vi "Vision_Right_R3.4.vi"() -> ()   [LabVIEW 2015]
uses:
  <vilib>/vision/driver/NI_Vision_Acquisition_Software.lvlib
  <vilib>/userdefined/High Color/IMAQdx.ctl
  <vilib>/vision/NI_Vision_Development_Module.lvlib
  <vilib>/vision/Pattern Matching.llb/IMAQ Match Range Setting.ctl
  <vilib>/vision/Pattern Matching.llb/IMAQ Curve Parameters.ctl
panel:
  in  "RIGHT ORIENTED\nSHARED VAR":bool
  out "LEFT ORIENTED\nSHARED VAR 2":bool
  out "STARTUP COMPLETE\nSHARED VAR":bool
  out "Facing South\nSHARED VAR":bool
  out "Found Template\nSHARED VAR":i32
  in  "StartCase Found - LEFT 2\nREAD SV":bool
  out "StartCase Found - LEFT\nSHARED VAR":bool
  in  "Min Corr Score\nStart":sgl
  out "Start Case\nCorrelation Score\nSHARED VAR":sgl
  in  "select (true= use advanced features\nfase= dont use) 2":bool
  in  "Start Template\nIndex":i32
  in  "Start Template \nFilePaths - ARRAY":path[](array[path])=[path "/home/lvuser/Beacon_Templates/Range_2/Sub 0 - Range 2.png", path "/home/lvuser/Beacon_Templates/Range_2/Sub 1 - Range 2.png", path "/home/lvuser/Beacon_Templates/Range_2/Sub 2 - Range 2.png", path "/home/lvuser/Beacon_Templates/Range_2/Sub 3 - Range 2.png", path "/home/lvuser/Beacon_Templates/Range_2/Sub 4 - Range 2.png"]
  in  "master Startup":bool=TRUE
  in  "Range 0 Default\nSetting Values":T1={"Min Scale"=50.0, "Max Scale"=160.0, "Min Score"=850.0, "Lower Transition Scale"=45.0, "Upper Transition Scale"=200.0, "ROI Vertical"=2.0, "ROI Horizontal"=1.0, "Scale Cushion"=15.0, "Curve Parameters"={"Min Length"=15, "Row Search Step"=10, "Col Search Step"=10}, "Beacon Cushion (px)"=3.0, "Max Scale Diff\nfrom Main"=50.0}
  in  "Range 0 Templates":T2={"Sub - 2 File Path"=path "/home/lvuser/Beacon_Templates/Range_0/Range 0.png", "Sub Beacon Template File Path - ARRAY"=[path "/home/lvuser/Beacon_Templates/Range_1/Sub 0 - Range 1.png", path "/home/lvuser/Beacon_Templates/Range_1/Sub 1 - Range 1.png", path "/home/lvuser/Beacon_Templates/Range_1/Sub 2 - Range 1.png", path "/home/lvuser/Beacon_Templates/Range_1/Sub 3 - Range 1.png", path "/home/lvuser/Beacon_Templates/Range_1/Sub 4 - Range 1.png"]}
  in  "Correlation Score Threhsold (Range 0)":sgl=750.0
  in  "stop":bool
  in  "select (true= use advanced features\nfase= dont use)":bool
  in  "Range 3 Default\nSetting Values":T1={"Min Scale"=50.0, "Max Scale"=150.0, "Min Score"=800.0, "Lower Transition Scale"=1.0, "Upper Transition Scale"=130.0, "ROI Vertical"=3.5, "ROI Horizontal"=4.0, "Scale Cushion"=15.0, "Curve Parameters"={"Min Length"=2, "Row Search Step"=5, "Col Search Step"=5}, "Beacon Cushion (px)"=5.0, "Max Scale Diff\nfrom Main"=10.0}
  in  "Range 2 Default\nSetting Values":T1={"Min Scale"=65.0, "Max Scale"=130.0, "Min Score"=800.0, "Lower Transition Scale"=65.0, "Upper Transition Scale"=125.0, "ROI Vertical"=2.8, "ROI Horizontal"=4.0, "Scale Cushion"=17.0, "Curve Parameters"={"Min Length"=10, "Row Search Step"=10, "Col Search Step"=10}, "Beacon Cushion (px)"=15.0, "Max Scale Diff\nfrom Main"=20.0}
  in  "No Lock Default\nSetting Values":T3={"Min Scale"=25.0, "Max Scale"=200.0, "Min Score"=750.0, "Lower Transition Scale"=35.0, "Upper Transition Scale"=250.0, "ROI Vertical"=15.0, "ROI Horizontal"=15.0, "Scale Cushion"=15.0, "Curve Parameters"={"Min Length"=5, "Row Search Step"=10, "Col Search Step"=10}, "Scale Cushion 2"=15.0, "Max Scale Diff\nfrom Main"=15.0}
  in  "ROI Decay Factor (px)":dbl=50.0
  in  "ROBOT STATE\n(fwd, bwd, neither) 2":i32
  in  "Score Decay \nFactor 2":dbl=50.0
  in  "Range 1 Default\nSetting Values":T1={"Min Scale"=25.0, "Max Scale"=100.0, "Min Score"=800.0, "Lower Transition Scale"=35.0, "Upper Transition Scale"=67.0, "ROI Vertical"=0.75, "ROI Horizontal"=5.0, "Scale Cushion"=23.0, "Curve Parameters"={"Min Length"=15, "Row Search Step"=15, "Col Search Step"=15}, "Beacon Cushion (px)"=25.0, "Max Scale Diff\nfrom Main"=25.0}
  out "Next Template":T4(ring)
  out "Current Template":T4(ring)
  in  "Initial Template":T4(ring)
  in  "Range 3 Templates":T2={"Sub - 2 File Path"=path "/home/lvuser/Beacon_Templates/Range_3/5 Beacons - Range 3.png", "Sub Beacon Template File Path - ARRAY"=[path "/home/lvuser/Beacon_Templates/Range_3/Sub 0 - Range 3.png", path "/home/lvuser/Beacon_Templates/Range_3/Sub 1 - Range 3.png", path "/home/lvuser/Beacon_Templates/Range_3/Sub 2 - Range 3.png", path "/home/lvuser/Beacon_Templates/Range_3/Sub 3 - Range 3.png", path "/home/lvuser/Beacon_Templates/Range_3/Sub 4 - Range 3.png"]}
  in  "Range 2 Templates":T2={"Sub - 2 File Path"=path "/home/lvuser/Beacon_Templates/Range_2/5 Beacons - Range 2.png", "Sub Beacon Template File Path - ARRAY"=[path "/home/lvuser/Beacon_Templates/Range_2/Sub 0 - Range 2.png", path "/home/lvuser/Beacon_Templates/Range_2/Sub 1 - Range 2.png", path "/home/lvuser/Beacon_Templates/Range_2/Sub 2 - Range 2.png", path "/home/lvuser/Beacon_Templates/Range_2/Sub 3 - Range 2.png", path "/home/lvuser/Beacon_Templates/Range_2/Sub 4 - Range 2.png"]}
  in  "Range 1 Templates - RIGHT":T2={"Sub - 2 File Path"=path "/home/lvuser/Beacon_Templates/Range_1/2_Beacons_Right - Range 1.png", "Sub Beacon Template File Path - ARRAY"=[path "/home/lvuser/Beacon_Templates/Range_1/Sub 0 - Range 1.png", path "/home/lvuser/Beacon_Templates/Range_1/Sub 1 - Range 1.png", path "/home/lvuser/Beacon_Templates/Range_1/Sub 2 - Range 1.png", path "/home/lvuser/Beacon_Templates/Range_1/Sub 3 - Range 1.png", path "/home/lvuser/Beacon_Templates/Range_1/Sub 4 - Range 1.png"]}
  out "Current Correlation Score":sgl
  in  "Correlation Score Threhsold":sgl=300.0
  out "New Min Score":dbl=800.0
  out "New Low Scale":dbl=25.0
  out "New high Scale":dbl=100.0
  in  "Absolute\nMinimum Score":dbl=750.0
  in  "Absolute\nMaximum Scale":dbl=250.0
  in  "Absolute\nMinimum Scale":dbl=25.0
  in  "Score\nCushion":dbl=192.0
  in  "Avg Scale - Last":dbl=50.0
  in  "Avg Score - Last":dbl=986.6820373535156
  in  "Max Window\n for Avg":u8=3
  in  "Valid Treshold\nfor Lock":i16=3
  out "Current  Score":sgl
  out "Current  Scale":sgl
  out "Current Valid?":bool
  out "Beacon - Scales":sgl[](array[numeric])
  out "beacon - Scores":sgl[](array[numeric])
  out "Beacons Found":bool[](array[boolean])
  out "Horiztonall Beacon \nCushion (pixels)":sgl=25.0
  out "Tracking Info":T5={"Lock"=FALSE, "Current Valid"=FALSE, "Current Template"=enum."Range 1", "Tracking Coordinates"={"X"=159.0, "Y"=119.0}, "Setting Values"={"Min Score"=800.0, "Min Scale"=25.0, "Max Scale"=100.0, "Curve Parameters"={"Min Length"=15, "Row Search Step"=15, "Col Search Step"=15}}}
  out "dT":u32=629
  out "Avg Scale":dbl=50.0
  out "Avg Score":dbl=986.6820373535156
  out "Current Search Settings":T8={"Curve Parameters"={"Extraction Mode"=1, "Edge Threshold"=200, "Edge Filter Size"=0, "Min Length"=15, "Row Search Step Size"=15, "Col Search Step Size"=15, "Max Endpoint Gap"=4, "Closed"=TRUE, "Subpixel"=TRUE}, "Match Mode"={"Rotation"=TRUE, "Scale"=TRUE, "Occlusion"=TRUE, "Reserved"=FALSE, "Reserved"=FALSE, "Reserved"=FALSE}, "Range Settings"=[{"Match Constraints"=0, "Min"=-10.0, "Max"=2.0}, {"Match Constraints"=1, "Min"=25.0, "Max"=100.0}, {"Match Constraints"=2, "Min"=0.0, "Max"=20.0}], "Number of Matches"=1, "Minimum Match Score"=800.0, "SubPixel Accuracy"=TRUE, "Adv. Geometric Match Options 2"=[{"Setup Data Item"=20, "Item Value"=0.0}, {"Setup Data Item"=22, "Item Value"=1.0}]} {"Curve Parameters"."Extraction Mode" items=["Normal", "Uniform Regions"]; "Curve Parameters"."Edge Filter Size" items=["Fine", "Normal", "Contour Tracing"]; "Curve Parameters"."Max Endpoint Gap" min=0; "Curve Parameters"."Col Search Step Size" min=1 max=255 step=1; "Curve Parameters"."Row Search Step Size" min=1 max=255 step=1; "Curve Parameters"."Min Length" min=0; "Curve Parameters"."Edge Threshold" min=1 max=350 step=1; "Range Settings"."Max" format="%.2f"; "Range Settings"."Min" format="%.2f"; "Range Settings"."Match Constraints" items=["Rotation Angle (degrees)", "Scale Factor (%)", "Occlusion (%)"]}
  out "Valid Scale History":dbl[](array[numeric]) format="%#_13g"
  out "Valid Score History":dbl[](array[numeric]) format="%#_13g"
  out "Valid Beacon History - in":bool[](array[boolean])
  out "Startup Flag":bool
  out "Lock Status":bool
  out "Y Coordinates":sgl[](array[numeric])
  out "X Coordinates":sgl[](array[numeric])
  out "Right Image out":T9(plugin-control)
  in  "History Size":i32=19
  in  "INITIAL Search Settings":T8={"Curve Parameters"={"Extraction Mode"=1, "Edge Threshold"=200, "Edge Filter Size"=0, "Min Length"=15, "Row Search Step Size"=10, "Col Search Step Size"=10, "Max Endpoint Gap"=4, "Closed"=TRUE, "Subpixel"=TRUE}, "Match Mode"={"Rotation"=TRUE, "Scale"=TRUE, "Occlusion"=TRUE, "Reserved"=FALSE, "Reserved"=FALSE, "Reserved"=FALSE}, "Range Settings"=[{"Match Constraints"=0, "Min"=-10.0, "Max"=2.0}, {"Match Constraints"=1, "Min"=25.0, "Max"=150.0}, {"Match Constraints"=2, "Min"=0.0, "Max"=20.0}], "Number of Matches"=1, "Minimum Match Score"=750.0, "SubPixel Accuracy"=TRUE, "Adv. Geometric Match Options 2"=[{"Setup Data Item"=20, "Item Value"=0.0}, {"Setup Data Item"=22, "Item Value"=1.0}]} {"Curve Parameters"."Extraction Mode" items=["Normal", "Uniform Regions"]; "Curve Parameters"."Edge Filter Size" items=["Fine", "Normal", "Contour Tracing"]; "Curve Parameters"."Max Endpoint Gap" min=0; "Curve Parameters"."Col Search Step Size" min=1 max=255 step=1; "Curve Parameters"."Row Search Step Size" min=1 max=255 step=1; "Curve Parameters"."Min Length" min=0; "Curve Parameters"."Edge Threshold" min=1 max=350 step=1; "Range Settings"."Max" format="%.2f"; "Range Settings"."Min" format="%.2f"; "Range Settings"."Match Constraints" items=["Rotation Angle (degrees)", "Scale Factor (%)", "Occlusion (%)"]; "Adv. Geometric Match Options 2"."Setup Data Item" items=["Curve Extraction Mode", "Curve Edge Threshold", "Curve Edge Filter Size", "Min Curve Length", "Curve Row Search Step Size", "Curve Col Search Step Size", "Curve Max Endpoint Gap", "Extract Closed Curves", "Enable Subpixel Curve Extraction", "Enable Correlation Score", "Enable Subpixel Accuracy", "Subpixel Iterations", "Subpixel Tolerance", "Initial Match List Length", "Enable Target Template Curve Score", "Min Match Separation Distance", "Min Match Separation Angle", "Min Match Separation Scale", "Max Match Overlap", "Enable Coarse Result", "Enable Calibration Support", "Enable Contrast Reversal", "Search Strategy", "Refinement Match Factor", "Subpixel Match Factor"]}
  # "ROI Factore (per Template)"
  # "Template Transition Scales"
  # "Search Parameter Limits"
  # "TEMPLATE FILE PATHS"
  # "Config"
  # "Initial Settings"
  # "STARTUP SPECIFIC"
  # "Range"
  # "Range"
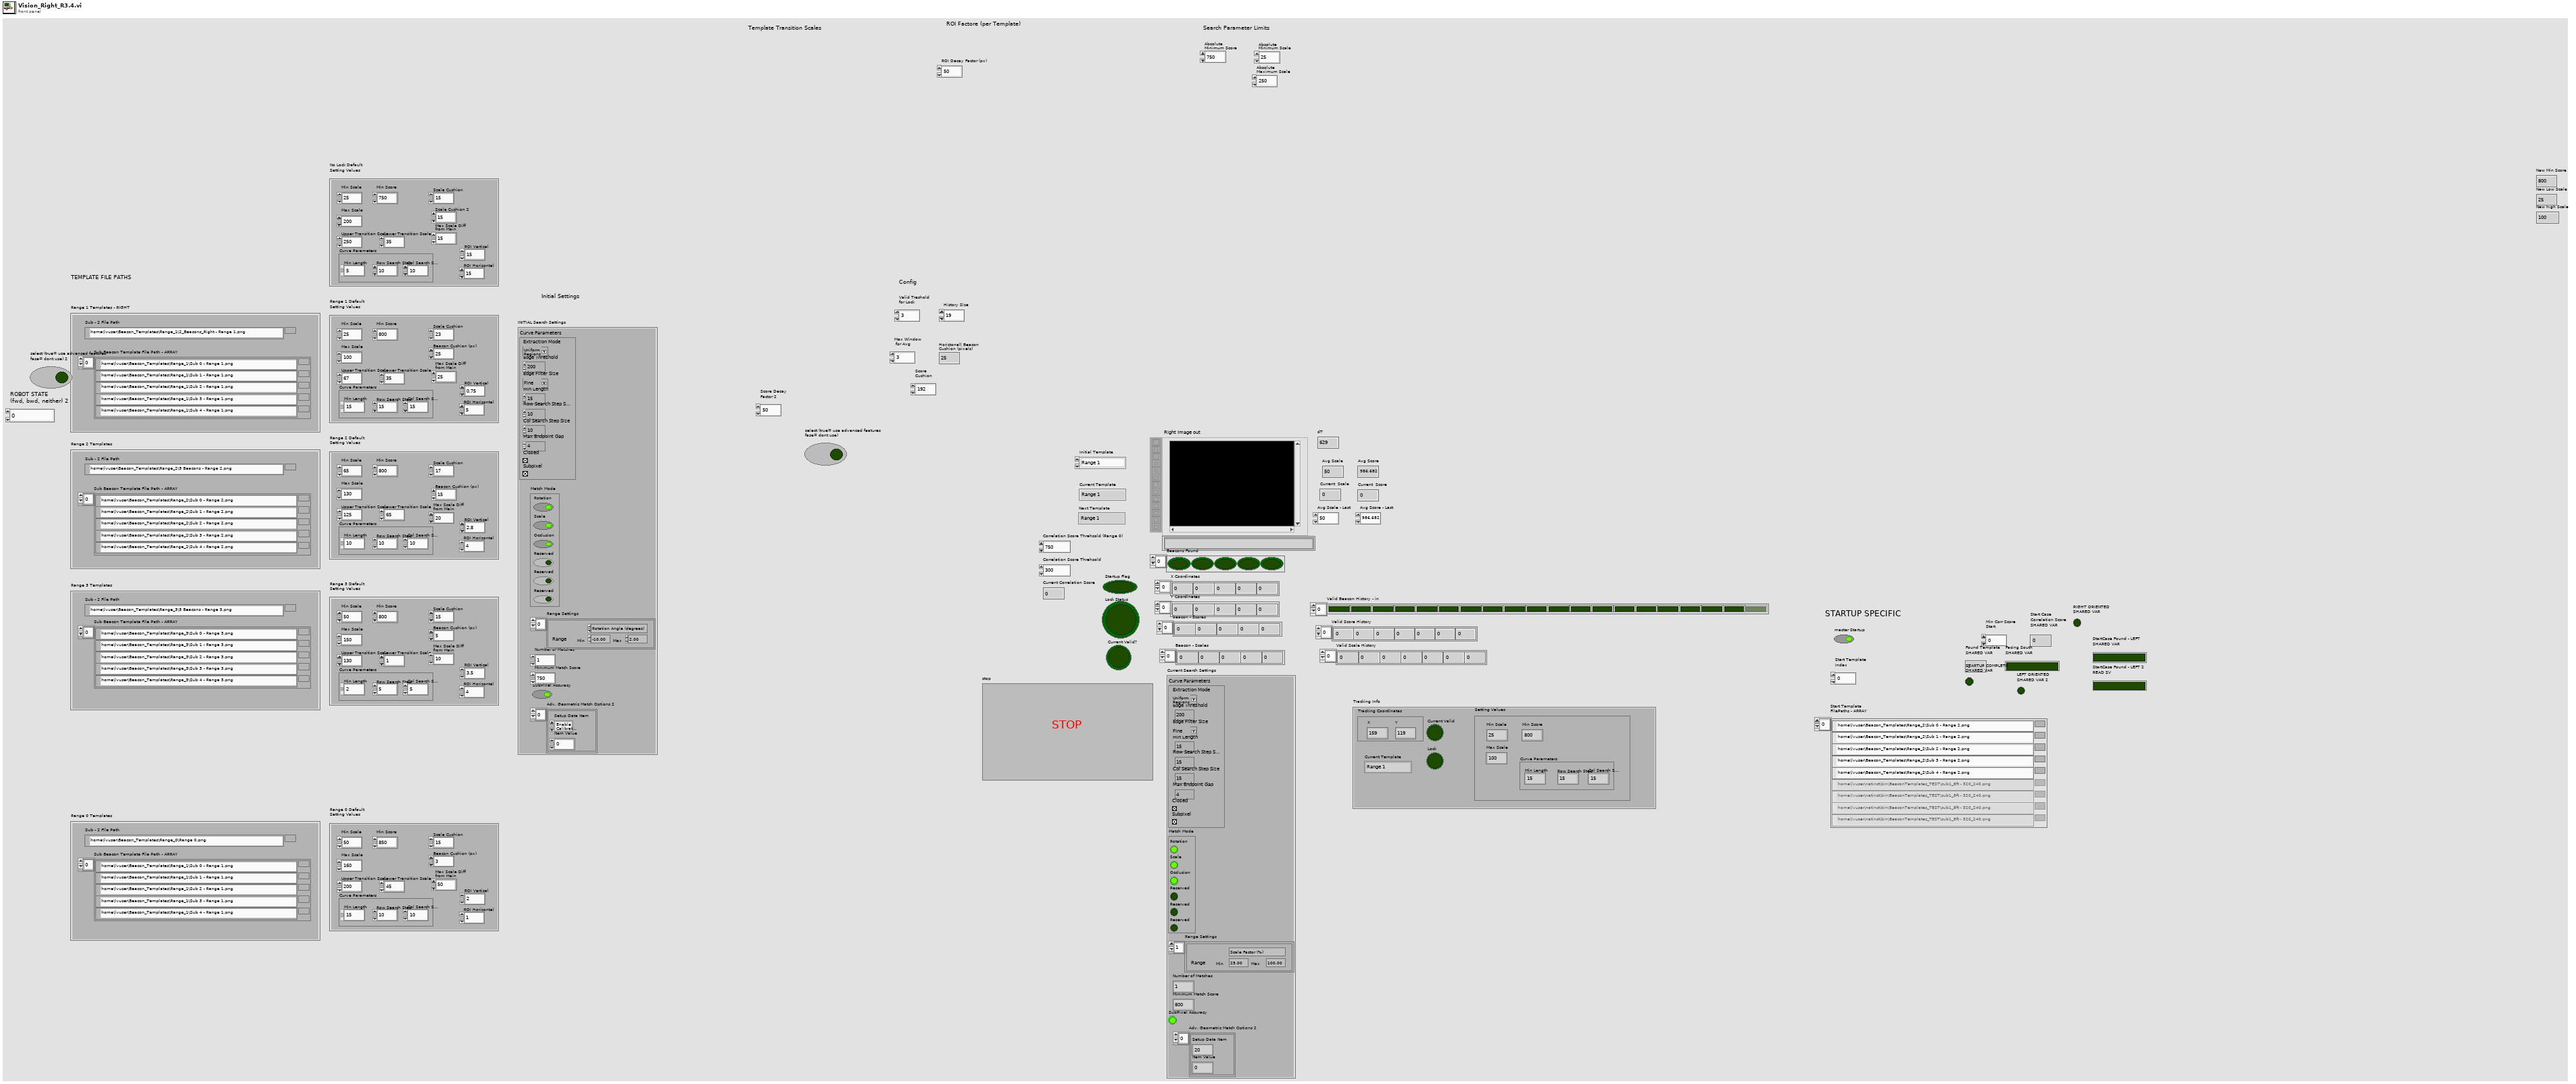
[diagram p1: front panel]
types:
  T1 = cluster{"Min Scale":dbl, "Max Scale":dbl, "Min Score":dbl, "Lower Transition Scale":sgl, "Upper Transition Scale":sgl, "ROI Vertical":dbl, "ROI Horizontal":dbl, "Scale Cushion":dbl, "Curve Parameters":cluster{"Min Length":i32, "Row Search Step":i32, "Col Search Step":i32}, "Beacon Cushion (px)":dbl, "Max Scale Diff\nfrom Main":dbl}
  T2 = cluster{"Sub - 2 File Path":path, "Sub Beacon Template File Path - ARRAY":path[]}
  T3 = cluster{"Min Scale":dbl, "Max Scale":dbl, "Min Score":dbl, "Lower Transition Scale":sgl, "Upper Transition Scale":sgl, "ROI Vertical":dbl, "ROI Horizontal":dbl, "Scale Cushion":dbl, "Curve Parameters":cluster{"Min Length":i32, "Row Search Step":i32, "Col Search Step":i32}, "Scale Cushion 2":dbl, "Max Scale Diff\nfrom Main":dbl}
  T4 = enum16{"Range 1", "Range 2", "Range 3", "Range 0"}
  T5 = cluster{"Lock":bool, "Current Valid":bool, "Current Template":enum16{"Range 1", "Range 2", "Range 3", "Range 0"}, "Tracking Coordinates":cluster{"X":dbl, "Y":dbl}, "Setting Values":cluster{"Min Score":dbl, "Min Scale":dbl, "Max Scale":dbl, "Curve Parameters":cluster{"Min Length":i32, "Row Search Step":i32, "Col Search Step":i32}}}
  T6 = typedef "IMAQ Curve Parameters.ctl" = cluster{"Extraction Mode":u32, "Edge Threshold":i32, "Edge Filter Size":u32, "Min Length":i32, "Row Search Step Size":i32, "Col Search Step Size":i32, "Max Endpoint Gap":i32, "Closed":bool, "Subpixel":bool}
  T7 = typedef "IMAQ Match Range Setting.ctl" = cluster{"Match Constraints":u32, "Min":dbl, "Max":dbl}
  T8 = cluster{"Curve Parameters":T6, "Match Mode":cluster{"Rotation":bool, "Scale":bool, "Occlusion":bool, "Reserved":bool, "Reserved":bool, "Reserved":bool}, "Range Settings":T7[], "Number of Matches":i32, "Minimum Match Score":sgl, "SubPixel Accuracy":bool, "Adv. Geometric Match Options 2":cluster{"Setup Data Item":u16, "Item Value":dbl}[]}
  T9 = typedef "IMAQ Image.ctl" = refnum<image>
  T10 = typedef "IMAQdx.ctl" = refnum<k21>
  T11 = typedef "Image Type" = u32
  T12 = typedef "ROI Descriptor" = cluster{"Global Rectangle":i32[], "Contours":cluster{"ID":enum32{"External", "Internal"}, "Type":u32, "Coordinates":i32[]}[]}
  T13 = cluster{"[0]":void, "[1]":void, "[2]":void, "[3]":void, "[4]":void, "[5]":void, "[6]":void, "[7]":void, "[8]":void}
  T14 = typedef "IMAQ GM Match Report.ctl" = cluster{"Position":cluster{"x":sgl, "y":sgl}, "Angle":sgl, "Scale":sgl, "Score":sgl, "Bounding Box":cluster{"x":sgl, "y":sgl}[], "Contrast Reversed":bool, "Occlusion %":sgl, "Template Target Curve Score":sgl, "Target Template Curve Score":sgl, "Correlation Score":sgl}
  T15 = cluster{"Matches[0]":T14, "Matches[1]":T14, "Matches[2]":T14, "Matches[3]":T14, "Matches[4]":T14, "Matches[5]":T14, "Matches[6]":T14, "Matches[7]":T14, "Matches[8]":T14}
  T16 = cluster{"Bounding Box[0]":cluster{"x":sgl, "y":sgl}, "Bounding Box[1]":cluster{"x":sgl, "y":sgl}, "Bounding Box[2]":cluster{"x":sgl, "y":sgl}, "Bounding Box[3]":cluster{"x":sgl, "y":sgl}, "Bounding Box[4]":cluster{"x":sgl, "y":sgl}, "Bounding Box[5]":cluster{"x":sgl, "y":sgl}, "Bounding Box[6]":cluster{"x":sgl, "y":sgl}, "Bounding Box[7]":cluster{"x":sgl, "y":sgl}, "Bounding Box[8]":cluster{"x":sgl, "y":sgl}}
  T17 = cluster{"Matches (Geometric Matching 1)[0]":T14, "Matches (Geometric Matching 1)[1]":T14, "Matches (Geometric Matching 1)[2]":T14, "Matches (Geometric Matching 1)[3]":T14, "Matches (Geometric Matching 1)[4]":T14, "Matches (Geometric Matching 1)[5]":T14, "Matches (Geometric Matching 1)[6]":T14, "Matches (Geometric Matching 1)[7]":T14, "Matches (Geometric Matching 1)[8]":T14}
  T18 = cluster{"Min Length":i32, "Row Search Step":i32, "Col Search Step":i32}
  T19 = cluster{"Extraction Mode":u32, "Edge Threshold":i32, "Edge Filter Size":u32, "Min Length":i32, "Row Search Step":i32, "Col Search Step":i32, "Max Endpoint Gap":i32, "Closed":bool, "Subpixel":bool}
  T20 = typedef "IMAQ Rectangle" = cluster{"Left":i32, "Top":i32, "Right":i32, "Bottom":i32, "Rotation":dbl}
  T21 = cluster{"Min Length":i32, "Row Search Step Size":i32, "Col Search Step Size":i32}
  T22 = cluster{"Min Score":dbl, "Min":dbl, "Max":dbl, cluster{"Min Length":i32, "Row Search Step Size":i32, "Col Search Step Size":i32}}
  T23 = cluster{bool, bool, "Initial Template":enum16{"Range 1", "Range 2", "Range 3", "Range 0"}, "Position":cluster{"x":dbl, "y":dbl}, cluster{"Min Score":dbl, "Min":dbl, "Max":dbl, cluster{"Min Length":i32, "Row Search Step Size":i32, "Col Search Step Size":i32}}}
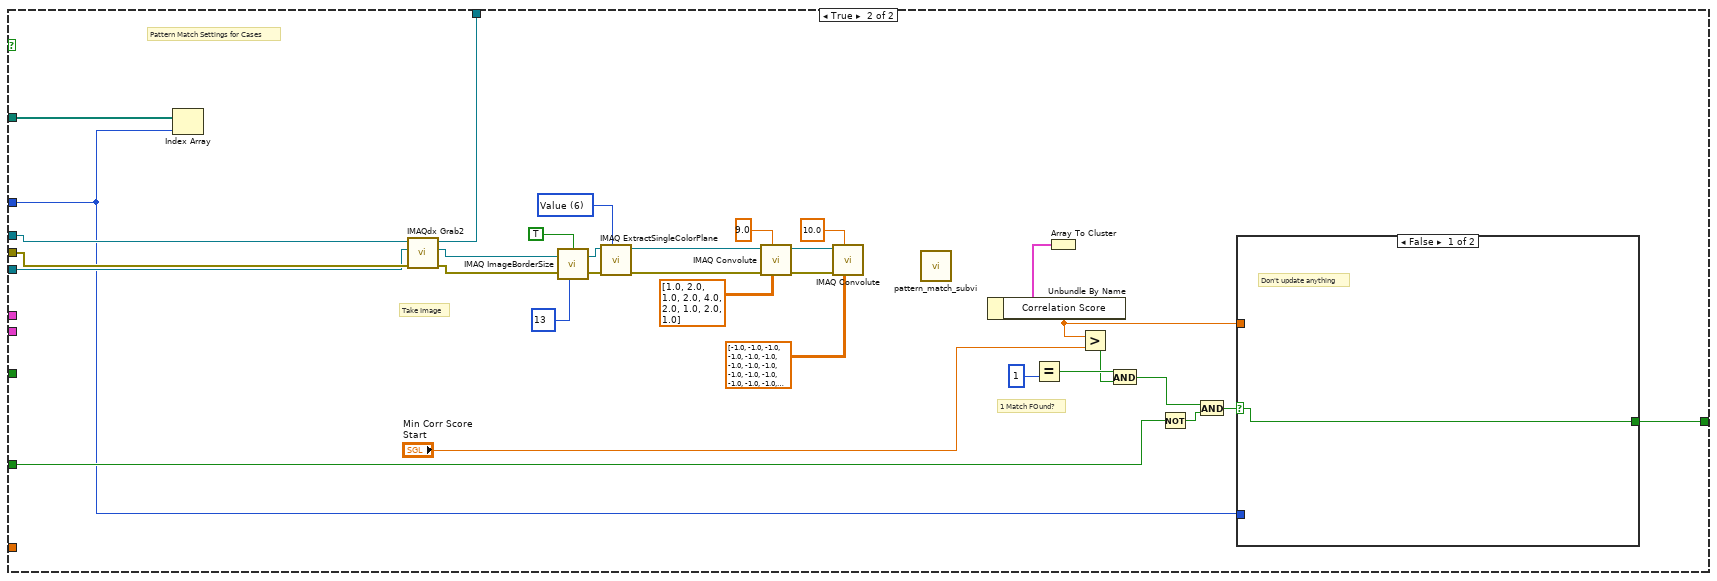
[diagram p2: hidden frame]
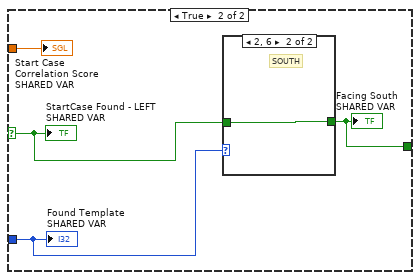
[diagram p3: hidden frame]
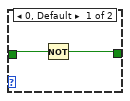
[diagram p4: hidden frame]
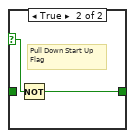
[diagram p5: hidden frame]
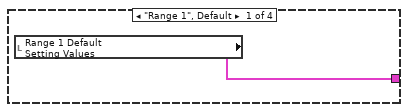
[diagram p6: hidden frame]
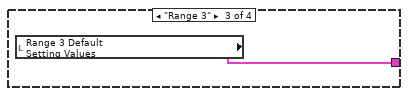
[diagram p7: hidden frame]
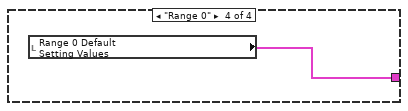
[diagram p8: hidden frame]
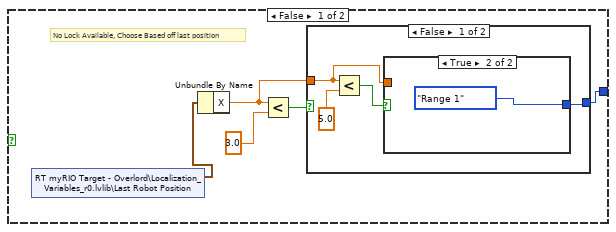
[diagram p9: hidden frame]
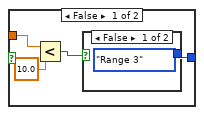
[diagram p10: hidden frame]
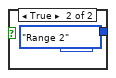
[diagram p11: hidden frame]
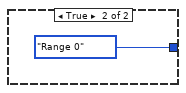
[diagram p12: hidden frame]
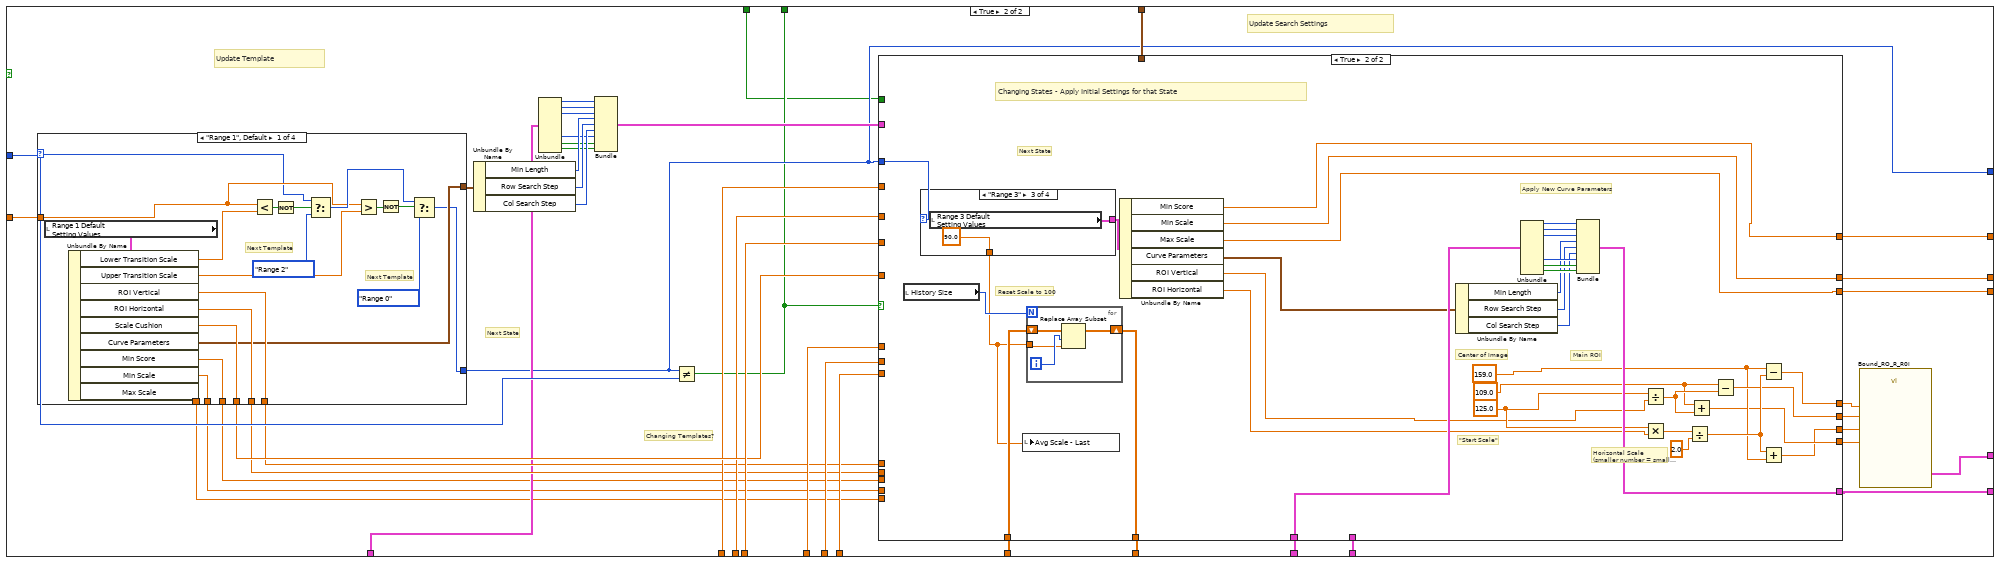
[diagram p13: hidden frame]
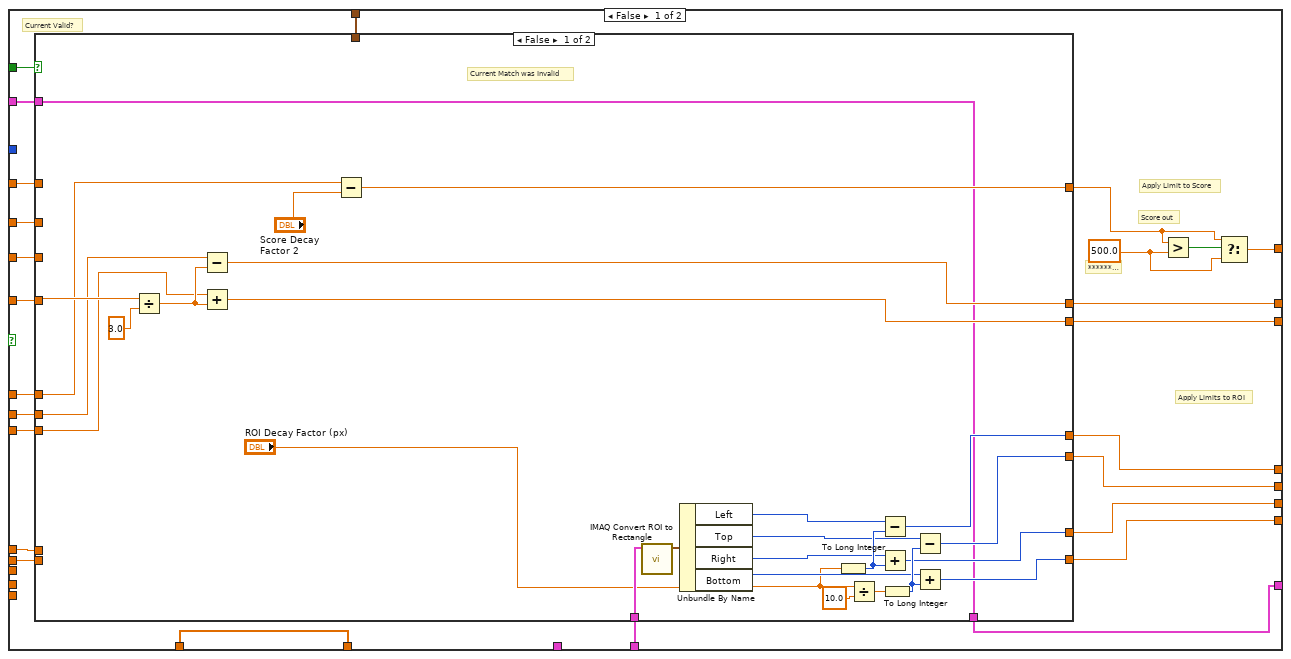
[diagram p14: hidden frame]
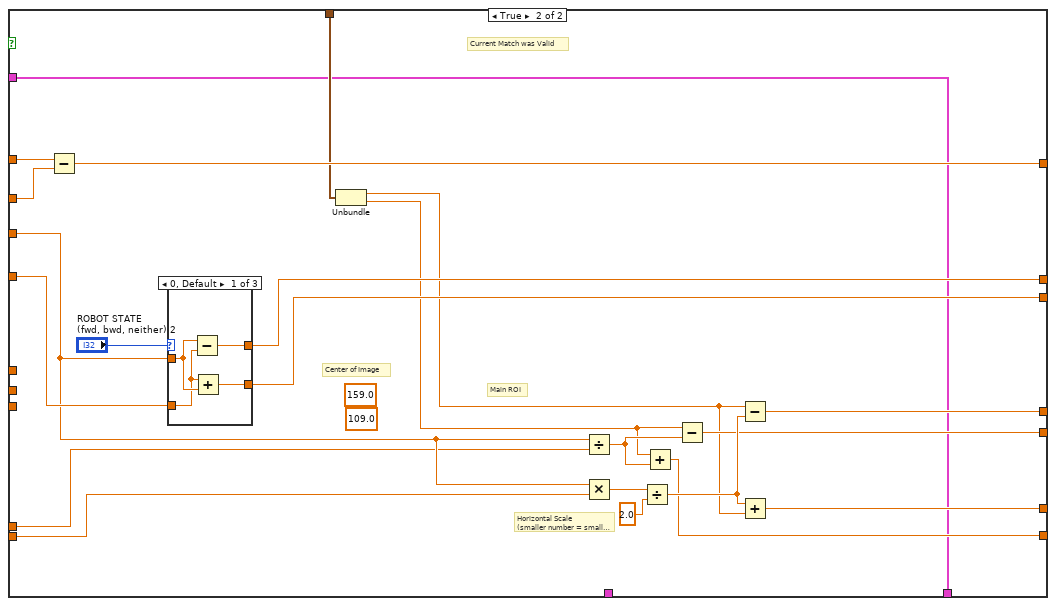
[diagram p15: hidden frame]
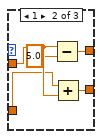
[diagram p16: hidden frame]
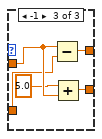
[diagram p17: hidden frame]
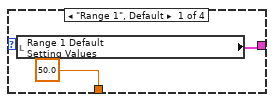
[diagram p18: hidden frame]
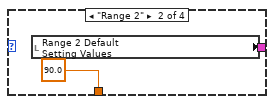
[diagram p19: hidden frame]
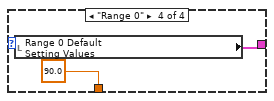
[diagram p20: hidden frame]
diagram:
  n1 = flat-sequence {
    tunnel: [w53] -> w30
    tunnel: ["INITIAL Search Settings"] -> w28
    tunnel: ["Initial Template"] -> w26
    tunnel: [TRUE] -> w24
    tunnel: [w50] -> w22
    tunnel: [w49] -> w20
    tunnel: [w48] -> w18
    tunnel: [w47] -> w16
    tunnel: [w46] -> w14
    tunnel: ["History Size"] -> w12
    tunnel: [750.0] -> w10
    tunnel: [100.0] -> w8
    tunnel: [w34] -> w6
    tunnel: [w33] -> w5
    tunnel: [w32] -> w3
    tunnel: w30 -> [w66]
    tunnel: [w66] -> w29
    tunnel: w28 -> [w65]
    tunnel: [w65] -> w27
    tunnel: w26 -> [w80]
    tunnel: [w80] -> w25
    tunnel: w24 -> [w79]
    tunnel: [w79] -> w23
    tunnel: w22 -> [w78]
    tunnel: [w78] -> w21
    tunnel: w20 -> [w77]
    tunnel: [w77] -> w19
    tunnel: w18 -> [w76]
    tunnel: [w76] -> w17
    tunnel: w16 -> [w75]
    tunnel: [w75] -> w15
    tunnel: w14 -> [w74]
    tunnel: [w74] -> w13
    tunnel: w12 -> [w73]
    tunnel: [w73] -> w11
    tunnel: w10 -> [w72]
    tunnel: [w72] -> w9
    tunnel: w8 -> [w71]
    tunnel: [w71] -> w7
    tunnel: w6 -> [w70]
    tunnel: w5 -> [w68]
    tunnel: [w68] -> w4
    tunnel: w3 -> [w69]
    tunnel: [w69] -> w2
    tunnel: [w67] -> w1
    tunnel: w29 -> [w183]
    tunnel: w27 -> [w182]
    tunnel: w25 -> [w181]
    tunnel: w23 -> [w180]
    tunnel: w21 -> [w176]
    tunnel: w19 -> [w173]
    tunnel: w17 -> [w179]
    tunnel: w15 -> [w178]
    tunnel: w13 -> [w177]
    tunnel: w11 -> [w175]
    tunnel: w9 -> [_]
    tunnel: w7 -> [_]
    tunnel: w4 -> [w171]
    tunnel: w2 -> [w170]
    tunnel: [w169] -> w31
    tunnel: w1 -> [w172]
    tunnel: w31 -> [w982]
    frame #0 {
      w39 = "[NIIMAQ_HEADER]\nType = 2\nVersion = 8\n\n[CAMERA_DATA]\nAcquisitionAttributes::Bayer::Algorithm = \"Bilinear\"\nAcquisitionAttributes::Bayer::GainB = \"1\"\nAcquisitionAttributes::Bayer::GainG = \"1\"\nAcquisitionAttributes::Bayer::GainR = \"1\"\nAcquisitionAttributes::Bayer::Pattern = \"Use hardware value\"\nAcquisitionAttributes::BitsPerPixel = \"Use hardware value\"\nAcquisitionAttributes::IgnoreFirstFrame = \"false\"\nAcquisitionAttributes::ImageDecoderCopyMode = \"Auto\"\nAcquisitionAttributes::OutputImageType = \"Auto\"\nAcquisitionAttributes::OverwriteMode = \"Get Newest\"\nAcquisitionAttributes::PixelSignedness = \"Use hardware value\"\nAcquisitionAttributes::ReceiveTimestampMode = \"None\"\nAcquisitionAttributes::ShiftPixelBits = \"false\"\nAcquisitionAttributes::SwapPixelBytes = \"false\"\nAcquisitionAttributes::Timeout = \"5000\"\nAcquisitionAttributes::VerticalMirror = \"false\"\nAcquisitionAttributes::VideoMode = \"320x240 YUY2 30.00fps\"\nCameraAttributes::BacklightCompensation::Mode = \"Manual\"\nCameraAttributes::BacklightCompensation::Value = \"false\"\nCameraAttributes::Brightness::Mode = \"UnknownEnumValue\"\nCameraAttributes::Brightness::Value = \"133\"\nCameraAttributes::Contrast::Mode = \"Manual\"\nCameraAttributes::Contrast::Value = \"0\"\nCameraAttributes::Exposure::Mode = \"Auto\"\nCameraAttributes::Focus::Mode = \"Auto\"\nCameraAttributes::Pan::Mode = \"Manual\"\nCameraAttributes::Pan::Value = \"0\"\nCameraAttributes::Saturation::Mode = \"Manual\"\nCameraAttributes::Saturation::Value = \"103\"\nCameraAttributes::Sharpness::Mode = \"Manual\"\nCameraAttributes::Sharpness::Value = \"25\"\nCameraAttributes::Tilt::Mode = \"Manual\"\nCameraAttributes::Tilt::Value = \"0\"\nCameraAttributes::WhiteBalance::Mode = \"Auto\"\nCameraAttributes::Zoom::Mode = \"Manual\"\nCameraAttributes::Zoom::Value = \"0\"\n"  # Attributes
      w60 = T11 0 items=["Grayscale (U8)", "Grayscale (I16)", "Grayscale (SGL)", "Complex (CSG)", "RGB (U32)", "HSL (U32)", "RGB (U64)", "Grayscale (U16)"] ("Image Type")
      # "avg start scale"
      # "Score History"
      # "Scale History"
      # "Valid Match History\n(main beacon)"
      # "Template State"
      # "Search Parameters"
      # "StartUp = True"
      # "Initial ROI Descriptor"
      # "INITIALIZE"
      n2 = call <vilib>:"IMAQdx Open Camera.vi"("Session In"=T10 "cam0") -> ("error out"=w37:errorcluster, "Session Out"=w38:T10)  [unwired: 2 in, 7 out]
      n3 = call <vilib>:"IMAQdx Read Attributes From String.vi"("error in"=w37, "Attributes String In"=w39, "Session In"=w38) -> ("error out"=w36:errorcluster, "Session Out"=w35:T10)  [unwired: 7 out]
      n4 = Bundle(0, 0, 640, 480, 0) -> (w59:cluster{i32, i32, i32, i32, i32})  [unwired: 1 in]
      n5 = call "IMAQ Convert Rectangle to ROI"("Rectangle"=w59) -> ("ROI Descriptor"=w53:T12)  [unwired: 8 in, 1 out]
      n6 = call "IMAQ Create"("Image Name"="Right_Image", "Image Type"=w60) -> ("New Image"=w50:T9, "error out"=w49:errorcluster)  [unwired: 3 in]
      n7 = Initialize Array(FALSE, "History Size") -> (w48:bool[])
      n8 = Initialize Array(0.0, "History Size") -> (w46:dbl[])
      n9 = Initialize Array(0.0, "History Size") -> (w47:dbl[])
      n10 = call <vilib>:"IMAQdx Configure Grab.vi"("error in"=w36, "Session In"=w35) -> ("error out"=w32:errorcluster, "Session Out"=w34:T10)  [unwired: 8 in]
      n11 = call "IMAQ Create"("Image Name"="Original") -> ("New Image"=w33:T9)  [unwired: 4 in, 1 out]
    }
    frame #1 {
      n12 = while {
        tunnel: w70 -> [w92]
        tunnel: w69 -> [w91]
        tunnel: w68 -> [w90]
        tunnel: [w89] -> w67
        tunnel: w66 -> [w85]
        tunnel: w65 -> [w84]
        stop <- w83 stop-if-true
        # "Shared Var"
        n13 = local read "Correlation Score Threhsold"() -> (w86:sgl)
        n14 = case shown="False" "master Startup" {
          tunnel: "Start Template\nIndex" -> [w99 w128]
          tunnel: "Start Template \nFilePaths - ARRAY" -> [_ w129]
          tunnel: w92 -> [w108 w160]
          tunnel: w91 -> [w106 w159]
          tunnel: w90 -> [w107 w158]
          tunnel: [w109 w141] -> w89
          tunnel: "StartCase Found - LEFT 2\nREAD SV" -> [_ w135]
          tunnel: "select (true= use advanced features\nfase= dont use) 2" -> [_ w130]
          tunnel: w86 -> [w100 _]
          tunnel: w85 -> [w98 _]
          tunnel: w84 -> [w97 _]
          tunnel: [w96 w126] -> w82
          frame False {
            w116 = 6 items=["Red", "Green", "Blue", "Hue", "Saturation", "Luminance", "Value", "Intensity"] ("Color Plane")
            # "1 Match FOund?"
            # "Take Image"
            n15 = call <vilib>:"IMAQdx Grab2.vi"("error in"=w106, "Image In"=w107, "Session In"=w108) -> ("error out"=w111:errorcluster, "Image Out"=w110:T9, "Session Out"=w109:T10)  [unwired: 5 in, 1 out]
            n16 = call "IMAQ ImageBorderSize"("Get/Set Status? (Set)"=TRUE, "Image"=w110, "Image border size in"=13 ("Border Size"), "error in (no error)"=w111) -> ("Image Out"=w117:T9, "error out"=w113:errorcluster)  [unwired: 1 out]
            n17 = call "IMAQ ExtractSingleColorPlane"("Color Plane"=w116, "error in (no error)"=w113, "Image Src"=w117) -> ("error out"=w118:errorcluster, "Image Dst Out"=w120:T9)  [unwired: 1 in, 6 out]
            n18 = call "IMAQ Convolute"("Kernel"=sgl[][] [[1.0, 2.0, 1.0], [2.0, 4.0, 2.0], [1.0, 2.0, 1.0]], "Divider (kernel sum)"=sgl 9.0 ("Divider"), "error in (no error)"=w118, "Image Src"=w120) -> ("error out"=w121:errorcluster, "Image Dst Out"=w124:T9)  [unwired: 3 in, 3 out]
            n19 = call "IMAQ Convolute"("Kernel"=sgl[][] [[-1.0, -1.0, -1.0, -1.0, -1.0, -1.0, -1.0, -1.0, -1.0, -1.0, -1.0, -1.0, -1.0, -1.0, -1.0, -1.0, -1.0, -1.0, -1.0, -1.0, -1.0, -1.0, -1.0, -1.0, -1.0, -1.0, -1.0], [-1.0, -1.0, -1.0, -1.0, -1.0, -1.0, -1.0, -1.0, -1.0, -1.0, -1.0, -1.0, -1.0, -1.0, -1.0, -1.0, -1.0, -1.0, -1.0, -1.0, -1.0, -1.0, -1.0, -1.0, -1.0, -1.0, -1.0], [-1.0, -1.0, -1.0, -1.0, -1.0, -1.0, -1.0, -1.0, -1.0, -1.0, -1.0, -1.0, -1.0, -1.0, -1.0, -1.0, -1.0, -1.0, -1.0, -1.0, -1.0, -1.0, -1.0, -1.0, -1.0, -1.0, -1.0], [-1.0, -1.0, -1.0, -1.0, -1.0, -1.0, -1.0, -1.0, -1.0, -1.0, -1.0, -1.0, -1.0, -1.0, -1.0, -1.0, -1.0, -1.0, -1.0, -1.0, -1.0, -1.0, -1.0, -1.0, -1.0, -1.0, -1.0], [-1.0, -1.0, -1.0, -1.0, -1.0, -1.0, -1.0, -1.0, -1.0, -1.0, -1.0, -1.0, -1.0, -1.0, -1.0, -1.0, -1.0, -1.0, -1.0, -1.0, -1.0, -1.0, -1.0, -1.0, -1.0, -1.0, -1.0], [-1.0, -1.0, -1.0, -1.0, -1.0, -1.0, -1.0, -1.0, -1.0, -1.0, -1.0, -1.0, -1.0, -1.0, -1.0, -1.0, -1.0, -1.0, -1.0, -1.0, -1.0, -1.0, -1.0, -1.0, -1.0, -1.0, -1.0], [-1.0, -1.0, -1.0, -1.0, -1.0, -1.0, -1.0, -1.0, -1.0, -1.0, -1.0, -1.0, -1.0, -1.0, -1.0, -1.0, -1.0, -1.0, -1.0, -1.0, -1.0, -1.0, -1.0, -1.0, -1.0, -1.0, -1.0], [-1.0, -1.0, -1.0, -1.0, -1.0, -1.0, -1.0, -1.0, -1.0, -1.0, -1.0, -1.0, -1.0, -1.0, -1.0, -1.0, -1.0, -1.0, -1.0, -1.0, -1.0, -1.0, -1.0, -1.0, -1.0, -1.0, -1.0], [-1.0, -1.0, -1.0, -1.0, -1.0, -1.0, -1.0, -1.0, -1.0, -1.0, -1.0, -1.0, -1.0, -1.0, -1.0, -1.0, -1.0, -1.0, -1.0, -1.0, -1.0, -1.0, -1.0, -1.0, -1.0, -1.0, -1.0], [-1.0, -1.0, -1.0, -1.0, -1.0, -1.0, -1.0, -1.0, -1.0, -1.0, -1.0, -1.0, -1.0, -1.0, -1.0, -1.0, -1.0, -1.0, -1.0, -1.0, -1.0, -1.0, -1.0, -1.0, -1.0, -1.0, -1.0], [-1.0, -1.0, -1.0, -1.0, -1.0, -1.0, -1.0, -1.0, -1.0, -1.0, -1.0, -1.0, -1.0, -1.0, -1.0, -1.0, -1.0, -1.0, -1.0, -1.0, -1.0, -1.0, -1.0, -1.0, -1.0, -1.0, -1.0], [-1.0, -1.0, -1.0, -1.0, -1.0, -1.0, -1.0, -1.0, -1.0, -1.0, -1.0, -1.0, -1.0, -1.0, -1.0, -1.0, -1.0, -1.0, -1.0, -1.0, -1.0, -1.0, -1.0, -1.0, -1.0, -1.0, -1.0], [-1.0, -1.0, -1.0, -1.0, -1.0, -1.0, -1.0, -1.0, -1.0, -1.0, -1.0, -1.0, -1.0, -1.0, -1.0, -1.0, -1.0, -1.0, -1.0, -1.0, -1.0, -1.0, -1.0, -1.0, -1.0, -1.0, -1.0], [-1.0, -1.0, -1.0, -1.0, -1.0, -1.0, -1.0, -1.0, -1.0, -1.0, -1.0, -1.0, -1.0, 728.0, -1.0, -1.0, -1.0, -1.0, -1.0, -1.0, -1.0, -1.0, -1.0, -1.0, -1.0, -1.0, -1.0], [-1.0, -1.0, -1.0, -1.0, -1.0, -1.0, -1.0, -1.0, -1.0, -1.0, -1.0, -1.0, -1.0, -1.0, -1.0, -1.0, -1.0, -1.0, -1.0, -1.0, -1.0, -1.0, -1.0, -1.0, -1.0, -1.0, -1.0], [-1.0, -1.0, -1.0, -1.0, -1.0, -1.0, -1.0, -1.0, -1.0, -1.0, -1.0, -1.0, -1.0, -1.0, -1.0, -1.0, -1.0, -1.0, -1.0, -1.0, -1.0, -1.0, -1.0, -1.0, -1.0, -1.0, -1.0], [-1.0, -1.0, -1.0, -1.0, -1.0, -1.0, -1.0, -1.0, -1.0, -1.0, -1.0, -1.0, -1.0, -1.0, -1.0, -1.0, -1.0, -1.0, -1.0, -1.0, -1.0, -1.0, -1.0, -1.0, -1.0, -1.0, -1.0], [-1.0, -1.0, -1.0, -1.0, -1.0, -1.0, -1.0, -1.0, -1.0, -1.0, -1.0, -1.0, -1.0, -1.0, -1.0, -1.0, -1.0, -1.0, -1.0, -1.0, -1.0, -1.0, -1.0, -1.0, -1.0, -1.0, -1.0], [-1.0, -1.0, -1.0, -1.0, -1.0, -1.0, -1.0, -1.0, -1.0, -1.0, -1.0, -1.0, -1.0, -1.0, -1.0, -1.0, -1.0, -1.0, -1.0, -1.0, -1.0, -1.0, -1.0, -1.0, -1.0, -1.0, -1.0], [-1.0, -1.0, -1.0, -1.0, -1.0, -1.0, -1.0, -1.0, -1.0, -1.0, -1.0, -1.0, -1.0, -1.0, -1.0, -1.0, -1.0, -1.0, -1.0, -1.0, -1.0, -1.0, -1.0, -1.0, -1.0, -1.0, -1.0], [-1.0, -1.0, -1.0, -1.0, -1.0, -1.0, -1.0, -1.0, -1.0, -1.0, -1.0, -1.0, -1.0, -1.0, -1.0, -1.0, -1.0, -1.0, -1.0, -1.0, -1.0, -1.0, -1.0, -1.0, -1.0, -1.0, -1.0], [-1.0, -1.0, -1.0, -1.0, -1.0, -1.0, -1.0, -1.0, -1.0, -1.0, -1.0, -1.0, -1.0, -1.0, -1.0, -1.0, -1.0, -1.0, -1.0, -1.0, -1.0, -1.0, -1.0, -1.0, -1.0, -1.0, -1.0], [-1.0, -1.0, -1.0, -1.0, -1.0, -1.0, -1.0, -1.0, -1.0, -1.0, -1.0, -1.0, -1.0, -1.0, -1.0, -1.0, -1.0, -1.0, -1.0, -1.0, -1.0, -1.0, -1.0, -1.0, -1.0, -1.0, -1.0], [-1.0, -1.0, -1.0, -1.0, -1.0, -1.0, -1.0, -1.0, -1.0, -1.0, -1.0, -1.0, -1.0, -1.0, -1.0, -1.0, -1.0, -1.0, -1.0, -1.0, -1.0, -1.0, -1.0, -1.0, -1.0, -1.0, -1.0], [-1.0, -1.0, -1.0, -1.0, -1.0, -1.0, -1.0, -1.0, -1.0, -1.0, -1.0, -1.0, -1.0, -1.0, -1.0, -1.0, -1.0, -1.0, -1.0, -1.0, -1.0, -1.0, -1.0, -1.0, -1.0, -1.0, -1.0], [-1.0, -1.0, -1.0, -1.0, -1.0, -1.0, -1.0, -1.0, -1.0, -1.0, -1.0, -1.0, -1.0, -1.0, -1.0, -1.0, -1.0, -1.0, -1.0, -1.0, -1.0, -1.0, -1.0, -1.0, -1.0, -1.0, -1.0], [-1.0, -1.0, -1.0, -1.0, -1.0, -1.0, -1.0, -1.0, -1.0, -1.0, -1.0, -1.0, -1.0, -1.0, -1.0, -1.0, -1.0, -1.0, -1.0, -1.0, -1.0, -1.0, -1.0, -1.0, -1.0, -1.0, -1.0]], "Divider (kernel sum)"=sgl 10.0 ("Divider"), "error in (no error)"=w121, "Image Src"=w124) -> ("error out"=w112:errorcluster)  [unwired: 3 in, 4 out]
            n20 = Equal?(y=1) -> (x = y?=w104:bool)  [unwired: 1 in]
            n21 = Array To Cluster() -> (cluster=w103:T13)  [unwired: 1 in]
            n22 = Unbundle By Name(w103) -> ("Correlation Score"=w101:sgl)
            n23 = Greater?(x=w101, y=w100) -> (0:w102:bool)
            n24 = And(x=w104, y=w102) -> (x .and. y?=w96:bool)
            "LEFT ORIENTED\nSHARED VAR 2" <- w96
          }
          frame True {
            w148 = 6 items=["Red", "Green", "Blue", "Hue", "Saturation", "Luminance", "Value", "Intensity"] ("Color Plane")
            # "Pattern Match Settings for Cases"
            # "1 Match FOund?"
            # "Take Image"
            n25 = Index Array(array=w129, index=w128) -> (element=w127:path)
            n26 = call <vilib>:"IMAQdx Grab2.vi"("error in"=w159, "Image In"=w158, "Session In"=w160) -> ("error out"=w143:errorcluster, "Image Out"=w142:T9, "Session Out"=w141:T10)  [unwired: 5 in, 1 out]
            n27 = call "IMAQ ImageBorderSize"("Get/Set Status? (Set)"=TRUE, "Image"=w142, "Image border size in"=13 ("Border Size"), "error in (no error)"=w143) -> ("Image Out"=w149:T9, "error out"=w145:errorcluster)  [unwired: 1 out]
            n28 = call "IMAQ ExtractSingleColorPlane"("Color Plane"=w148, "error in (no error)"=w145, "Image Src"=w149) -> ("error out"=w150:errorcluster, "Image Dst Out"=w152:T9)  [unwired: 1 in, 6 out]
            n29 = call "IMAQ Convolute"("Kernel"=sgl[][] [[1.0, 2.0, 1.0], [2.0, 4.0, 2.0], [1.0, 2.0, 1.0]], "Divider (kernel sum)"=sgl 9.0 ("Divider"), "error in (no error)"=w150, "Image Src"=w152) -> ("error out"=w153:errorcluster, "Image Dst Out"=w156:T9)  [unwired: 3 in, 3 out]
            n30 = call "IMAQ Convolute"("Kernel"=sgl[][] [[-1.0, -1.0, -1.0, -1.0, -1.0, -1.0, -1.0, -1.0, -1.0, -1.0, -1.0, -1.0, -1.0, -1.0, -1.0, -1.0, -1.0, -1.0, -1.0, -1.0, -1.0, -1.0, -1.0, -1.0, -1.0, -1.0, -1.0], [-1.0, -1.0, -1.0, -1.0, -1.0, -1.0, -1.0, -1.0, -1.0, -1.0, -1.0, -1.0, -1.0, -1.0, -1.0, -1.0, -1.0, -1.0, -1.0, -1.0, -1.0, -1.0, -1.0, -1.0, -1.0, -1.0, -1.0], [-1.0, -1.0, -1.0, -1.0, -1.0, -1.0, -1.0, -1.0, -1.0, -1.0, -1.0, -1.0, -1.0, -1.0, -1.0, -1.0, -1.0, -1.0, -1.0, -1.0, -1.0, -1.0, -1.0, -1.0, -1.0, -1.0, -1.0], [-1.0, -1.0, -1.0, -1.0, -1.0, -1.0, -1.0, -1.0, -1.0, -1.0, -1.0, -1.0, -1.0, -1.0, -1.0, -1.0, -1.0, -1.0, -1.0, -1.0, -1.0, -1.0, -1.0, -1.0, -1.0, -1.0, -1.0], [-1.0, -1.0, -1.0, -1.0, -1.0, -1.0, -1.0, -1.0, -1.0, -1.0, -1.0, -1.0, -1.0, -1.0, -1.0, -1.0, -1.0, -1.0, -1.0, -1.0, -1.0, -1.0, -1.0, -1.0, -1.0, -1.0, -1.0], [-1.0, -1.0, -1.0, -1.0, -1.0, -1.0, -1.0, -1.0, -1.0, -1.0, -1.0, -1.0, -1.0, -1.0, -1.0, -1.0, -1.0, -1.0, -1.0, -1.0, -1.0, -1.0, -1.0, -1.0, -1.0, -1.0, -1.0], [-1.0, -1.0, -1.0, -1.0, -1.0, -1.0, -1.0, -1.0, -1.0, -1.0, -1.0, -1.0, -1.0, -1.0, -1.0, -1.0, -1.0, -1.0, -1.0, -1.0, -1.0, -1.0, -1.0, -1.0, -1.0, -1.0, -1.0], [-1.0, -1.0, -1.0, -1.0, -1.0, -1.0, -1.0, -1.0, -1.0, -1.0, -1.0, -1.0, -1.0, -1.0, -1.0, -1.0, -1.0, -1.0, -1.0, -1.0, -1.0, -1.0, -1.0, -1.0, -1.0, -1.0, -1.0], [-1.0, -1.0, -1.0, -1.0, -1.0, -1.0, -1.0, -1.0, -1.0, -1.0, -1.0, -1.0, -1.0, -1.0, -1.0, -1.0, -1.0, -1.0, -1.0, -1.0, -1.0, -1.0, -1.0, -1.0, -1.0, -1.0, -1.0], [-1.0, -1.0, -1.0, -1.0, -1.0, -1.0, -1.0, -1.0, -1.0, -1.0, -1.0, -1.0, -1.0, -1.0, -1.0, -1.0, -1.0, -1.0, -1.0, -1.0, -1.0, -1.0, -1.0, -1.0, -1.0, -1.0, -1.0], [-1.0, -1.0, -1.0, -1.0, -1.0, -1.0, -1.0, -1.0, -1.0, -1.0, -1.0, -1.0, -1.0, -1.0, -1.0, -1.0, -1.0, -1.0, -1.0, -1.0, -1.0, -1.0, -1.0, -1.0, -1.0, -1.0, -1.0], [-1.0, -1.0, -1.0, -1.0, -1.0, -1.0, -1.0, -1.0, -1.0, -1.0, -1.0, -1.0, -1.0, -1.0, -1.0, -1.0, -1.0, -1.0, -1.0, -1.0, -1.0, -1.0, -1.0, -1.0, -1.0, -1.0, -1.0], [-1.0, -1.0, -1.0, -1.0, -1.0, -1.0, -1.0, -1.0, -1.0, -1.0, -1.0, -1.0, -1.0, -1.0, -1.0, -1.0, -1.0, -1.0, -1.0, -1.0, -1.0, -1.0, -1.0, -1.0, -1.0, -1.0, -1.0], [-1.0, -1.0, -1.0, -1.0, -1.0, -1.0, -1.0, -1.0, -1.0, -1.0, -1.0, -1.0, -1.0, 728.0, -1.0, -1.0, -1.0, -1.0, -1.0, -1.0, -1.0, -1.0, -1.0, -1.0, -1.0, -1.0, -1.0], [-1.0, -1.0, -1.0, -1.0, -1.0, -1.0, -1.0, -1.0, -1.0, -1.0, -1.0, -1.0, -1.0, -1.0, -1.0, -1.0, -1.0, -1.0, -1.0, -1.0, -1.0, -1.0, -1.0, -1.0, -1.0, -1.0, -1.0], [-1.0, -1.0, -1.0, -1.0, -1.0, -1.0, -1.0, -1.0, -1.0, -1.0, -1.0, -1.0, -1.0, -1.0, -1.0, -1.0, -1.0, -1.0, -1.0, -1.0, -1.0, -1.0, -1.0, -1.0, -1.0, -1.0, -1.0], [-1.0, -1.0, -1.0, -1.0, -1.0, -1.0, -1.0, -1.0, -1.0, -1.0, -1.0, -1.0, -1.0, -1.0, -1.0, -1.0, -1.0, -1.0, -1.0, -1.0, -1.0, -1.0, -1.0, -1.0, -1.0, -1.0, -1.0], [-1.0, -1.0, -1.0, -1.0, -1.0, -1.0, -1.0, -1.0, -1.0, -1.0, -1.0, -1.0, -1.0, -1.0, -1.0, -1.0, -1.0, -1.0, -1.0, -1.0, -1.0, -1.0, -1.0, -1.0, -1.0, -1.0, -1.0], [-1.0, -1.0, -1.0, -1.0, -1.0, -1.0, -1.0, -1.0, -1.0, -1.0, -1.0, -1.0, -1.0, -1.0, -1.0, -1.0, -1.0, -1.0, -1.0, -1.0, -1.0, -1.0, -1.0, -1.0, -1.0, -1.0, -1.0], [-1.0, -1.0, -1.0, -1.0, -1.0, -1.0, -1.0, -1.0, -1.0, -1.0, -1.0, -1.0, -1.0, -1.0, -1.0, -1.0, -1.0, -1.0, -1.0, -1.0, -1.0, -1.0, -1.0, -1.0, -1.0, -1.0, -1.0], [-1.0, -1.0, -1.0, -1.0, -1.0, -1.0, -1.0, -1.0, -1.0, -1.0, -1.0, -1.0, -1.0, -1.0, -1.0, -1.0, -1.0, -1.0, -1.0, -1.0, -1.0, -1.0, -1.0, -1.0, -1.0, -1.0, -1.0], [-1.0, -1.0, -1.0, -1.0, -1.0, -1.0, -1.0, -1.0, -1.0, -1.0, -1.0, -1.0, -1.0, -1.0, -1.0, -1.0, -1.0, -1.0, -1.0, -1.0, -1.0, -1.0, -1.0, -1.0, -1.0, -1.0, -1.0], [-1.0, -1.0, -1.0, -1.0, -1.0, -1.0, -1.0, -1.0, -1.0, -1.0, -1.0, -1.0, -1.0, -1.0, -1.0, -1.0, -1.0, -1.0, -1.0, -1.0, -1.0, -1.0, -1.0, -1.0, -1.0, -1.0, -1.0], [-1.0, -1.0, -1.0, -1.0, -1.0, -1.0, -1.0, -1.0, -1.0, -1.0, -1.0, -1.0, -1.0, -1.0, -1.0, -1.0, -1.0, -1.0, -1.0, -1.0, -1.0, -1.0, -1.0, -1.0, -1.0, -1.0, -1.0], [-1.0, -1.0, -1.0, -1.0, -1.0, -1.0, -1.0, -1.0, -1.0, -1.0, -1.0, -1.0, -1.0, -1.0, -1.0, -1.0, -1.0, -1.0, -1.0, -1.0, -1.0, -1.0, -1.0, -1.0, -1.0, -1.0, -1.0], [-1.0, -1.0, -1.0, -1.0, -1.0, -1.0, -1.0, -1.0, -1.0, -1.0, -1.0, -1.0, -1.0, -1.0, -1.0, -1.0, -1.0, -1.0, -1.0, -1.0, -1.0, -1.0, -1.0, -1.0, -1.0, -1.0, -1.0], [-1.0, -1.0, -1.0, -1.0, -1.0, -1.0, -1.0, -1.0, -1.0, -1.0, -1.0, -1.0, -1.0, -1.0, -1.0, -1.0, -1.0, -1.0, -1.0, -1.0, -1.0, -1.0, -1.0, -1.0, -1.0, -1.0, -1.0]], "Divider (kernel sum)"=sgl 10.0 ("Divider"), "error in (no error)"=w153, "Image Src"=w156) -> ("error out"=w144:errorcluster)  [unwired: 3 in, 4 out]
            n31 = call "pattern_match_subvi.vi"() -> ()  [unwired: 12 in, 4 out]
            n32 = Equal?(y=1) -> (x = y?=w139:bool)  [unwired: 1 in]
            n33 = Array To Cluster() -> (cluster=w138:T13)  [unwired: 1 in]
            n34 = Unbundle By Name(w138) -> ("Correlation Score"=w131:sgl)
            n35 = Greater?(x=w131, y="Min Corr Score\nStart") -> (0:w137:bool)
            n36 = And(x=w139, y=w137) -> (x .and. y?=w132:bool)
            n37 = Not(x=w135) -> (.not. x?=w133:bool)
            n38 = And(x=w132, y=w133) -> (x .and. y?=w134:bool)
            n39 = case shown="False" w134 {
              selector: w134 -> [w161 w163]
              tunnel: w131 -> [_ w165]
              tunnel: w128 -> [_ w164]
              tunnel: [w161 w162] -> w126
              frame False {
                # "Don't update anything"
              }
              frame True {
                n40 = case shown="2, 6" w164 {
                  tunnel: w163 -> [w167 w168]
                  tunnel: [w166 w168] -> w162
                  frame 0, Default {
                    n41 = Not(x=w167) -> (.not. x?=w166:bool)
                  }
                  frame 2, 6 {
                    # "SOUTH"
                  }
                }
                "Facing South\nSHARED VAR" <- w162
                "Start Case\nCorrelation Score\nSHARED VAR" <- w165
                "StartCase Found - LEFT\nSHARED VAR" <- w163
                "Found Template\nSHARED VAR" <- w164
              }
            }
          }
        }
        "STARTUP COMPLETE\nSHARED VAR" <- w82
        n42 = Or(x=w82, y="RIGHT ORIENTED\nSHARED VAR") -> (x .or. y?=w83:bool)
      }
    }
    frame #2 {
      # "Avg Scale"
      # "Avg Score"
      # "Score History"
      # "Scale History"
      # "Valid Match History\n(main beacon)"
      # "Sub Beacon Search Array"
      # "StartUp = True"
      # "Template State"
      # "Search Parameters"
      # "ROI"
      n43 = call "Tick Count"() -> ("Tick Count(mSec)"=w174:u32)
      n44 = while {
        shift-right: [w196] -> _
        shift-left: w183 -> [w210]
        shift-right: [w206] -> _
        shift-left: w182 -> [w211]
        shift-right: [w195] -> _
        shift-left: w181 -> [w198]
        shift-right: [w193] -> _
        shift-left: w180 -> [w194]
        shift-right: [w202] -> _
        shift-left: w179 -> [w203]
        shift-right: [w192] -> _
        shift-left: w178 -> [w201]
        shift-right: [w199] -> _
        shift-left: w177 -> [w200]
        shift-right: [w205] -> _
        shift-left: w176 -> [w212]
        tunnel: w175 -> [w217]
        shift-right: [w215] -> _
        shift-left: w174 -> [w216]
        tunnel: w173 -> [w204]
        tunnel: w172 -> [w191]
        tunnel: w171 -> [w190]
        tunnel: w170 -> [w189]
        tunnel: [w186] -> w169
        stop <- "stop" stop-if-true
        n45 = call "Tick Count2"() -> ("Tick Count(mSec)"=w215:u32)
        n46 = Subtract(x=w215, y=w216) -> (x-y=→"dT":u32)
        n47 = flat-sequence {
          tunnel: [w218] -> w208
          tunnel: [w225] -> w213
          tunnel: w212 -> [w225]
          tunnel: [w225] -> w205
          tunnel: w204 -> [_]
          tunnel: w191 -> [w224]
          tunnel: w190 -> [w223]
          tunnel: w189 -> [w222]
          tunnel: [w221] -> w188
          tunnel: [w220] -> w187
          tunnel: [w219] -> w185
          tunnel: w198 -> [w236]
          tunnel: w203 -> [w343]
          tunnel: w201 -> [w342]
          tunnel: w200 -> [w341]
          tunnel: w217 -> [_]
          tunnel: w213 -> [w247]
          tunnel: w211 -> [w248]
          tunnel: w210 -> [w250]
          tunnel: [w310] -> w209
          tunnel: w208 -> [w303]
          tunnel: [w303] -> w207
          tunnel: [w302] -> w202
          tunnel: [w270] -> _
          tunnel: [w301] -> w199
          tunnel: w194 -> [w268]
          tunnel: [w272] -> w197
          tunnel: [w273] -> w196
          tunnel: [w272] -> w195
          tunnel: [w267] -> w193
          tunnel: [w271] -> w192
          tunnel: w188 -> [w242]
          tunnel: w187 -> [w241]
          tunnel: [w240] -> w186
          tunnel: w185 -> [w240]
          tunnel: w209 -> [w981]
          tunnel: w207 -> [w979]
          tunnel: [w981] -> w206
          tunnel: [w980] -> _
          tunnel: w197 -> [w980]
          frame #0 {
            # "Aquire Image"
            n48 = shared-variable "RT myRIO Target - Overlord\\Localization_Variables_r0.lvlib\\Right Servo Angle_Current"() -> (w218:dbl)  [unwired: 1 in, 1 out]
            n49 = call <vilib>:"IMAQdx Grab2.vi"("error in"=w222, "Image In"=w223, "Session In"=w224) -> ("error out"=w220:errorcluster, "Image Out"=w221:T9, "Session Out"=w219:T10)  [unwired: 5 in, 1 out]
          }
          frame #1 {
            (unwired) T4."Range 1" ("Initial Template 2")
            w260 = 6 items=["Red", "Green", "Blue", "Hue", "Saturation", "Luminance", "Value", "Intensity"] ("Color Plane")
            w313 = u32 1 ("index")
            # "Tracking Position"
            # "ROI center"
            # "Add mode when CLose to look for all individual beacons with full ROI"
            # "Service Start Up Flag"
            # "Change States?"
            # "Next Template"
            # "Max Scale"
            # "Min Scale"
            # "Min Score"
            # "Curve p"
            # "ROI"
            # "Current Scale Range"
            # "Current Min Score"
            # "Avg Score"
            # "Avg Scale"
            # "Startup?"
            # "********** Look into False case **********"
            # "SUm # of Sub-Beacons Found, Check if Enoough\nto be considered Valid"
            # "Update Tracking Coordinates"
            # "Next Settings"
            # "Current Settings"
            # "Current Min\n& Max Scale"
            # "Scale"
            # "Min Score"
            # "Lower Scale"
            # "Upper Scale"
            # "Min Score out"
            # "Score History"
            # "Min Required to use avarage"
            # "Scale History"
            # "History Size"
            # "Calculate Average Score/Scale"
            # "****# of previous in history that must be true\nin order for position to be considered \"locked\""
            # "Scale History"
            # "Score History"
            # "Valid History"
            # "Update History Data"
            # "1 Match FOund?"
            # "# of Sub Beacons"
            # "Sub Beacons to Search For"
            # "# Sub Beacons to Find in\norder to be valid"
            # "Template Filepath & Sub Beacon Array"
            # "Select Current Template Config"
            # "Pattern Match to Current Template"
            # "Apply FIltering"
            n50 = call "IMAQ ImageBorderSize"("Get/Set Status? (Set)"=TRUE, "Image"=w242, "Image border size in"=13 ("Border Size"), "error in (no error)"=w241) -> ("Image Out"=w259:T9, "error out"=w263:errorcluster)  [unwired: 1 out]
            n51 = call "IMAQ ExtractSingleColorPlane"("Color Plane"=w260, "error in (no error)"=w263, "Image Src"=w259) -> ("error out"=w258:errorcluster, "Image Dst Out"=w256:T9)  [unwired: 1 in, 6 out]
            n52 = call "IMAQ Convolute"("Kernel"=sgl[][] [[1.0, 2.0, 1.0], [2.0, 4.0, 2.0], [1.0, 2.0, 1.0]], "Divider (kernel sum)"=sgl 9.0 ("Divider"), "error in (no error)"=w258, "Image Src"=w256) -> ("error out"=w255:errorcluster, "Image Dst Out"=w252:T9)  [unwired: 3 in, 3 out]
            n53 = call "IMAQ Convolute"("Kernel"=sgl[][] [[-1.0, -1.0, -1.0, -1.0, -1.0, -1.0, -1.0, -1.0, -1.0, -1.0, -1.0, -1.0, -1.0, -1.0, -1.0, -1.0, -1.0, -1.0, -1.0, -1.0, -1.0, -1.0, -1.0, -1.0, -1.0, -1.0, -1.0], [-1.0, -1.0, -1.0, -1.0, -1.0, -1.0, -1.0, -1.0, -1.0, -1.0, -1.0, -1.0, -1.0, -1.0, -1.0, -1.0, -1.0, -1.0, -1.0, -1.0, -1.0, -1.0, -1.0, -1.0, -1.0, -1.0, -1.0], [-1.0, -1.0, -1.0, -1.0, -1.0, -1.0, -1.0, -1.0, -1.0, -1.0, -1.0, -1.0, -1.0, -1.0, -1.0, -1.0, -1.0, -1.0, -1.0, -1.0, -1.0, -1.0, -1.0, -1.0, -1.0, -1.0, -1.0], [-1.0, -1.0, -1.0, -1.0, -1.0, -1.0, -1.0, -1.0, -1.0, -1.0, -1.0, -1.0, -1.0, -1.0, -1.0, -1.0, -1.0, -1.0, -1.0, -1.0, -1.0, -1.0, -1.0, -1.0, -1.0, -1.0, -1.0], [-1.0, -1.0, -1.0, -1.0, -1.0, -1.0, -1.0, -1.0, -1.0, -1.0, -1.0, -1.0, -1.0, -1.0, -1.0, -1.0, -1.0, -1.0, -1.0, -1.0, -1.0, -1.0, -1.0, -1.0, -1.0, -1.0, -1.0], [-1.0, -1.0, -1.0, -1.0, -1.0, -1.0, -1.0, -1.0, -1.0, -1.0, -1.0, -1.0, -1.0, -1.0, -1.0, -1.0, -1.0, -1.0, -1.0, -1.0, -1.0, -1.0, -1.0, -1.0, -1.0, -1.0, -1.0], [-1.0, -1.0, -1.0, -1.0, -1.0, -1.0, -1.0, -1.0, -1.0, -1.0, -1.0, -1.0, -1.0, -1.0, -1.0, -1.0, -1.0, -1.0, -1.0, -1.0, -1.0, -1.0, -1.0, -1.0, -1.0, -1.0, -1.0], [-1.0, -1.0, -1.0, -1.0, -1.0, -1.0, -1.0, -1.0, -1.0, -1.0, -1.0, -1.0, -1.0, -1.0, -1.0, -1.0, -1.0, -1.0, -1.0, -1.0, -1.0, -1.0, -1.0, -1.0, -1.0, -1.0, -1.0], [-1.0, -1.0, -1.0, -1.0, -1.0, -1.0, -1.0, -1.0, -1.0, -1.0, -1.0, -1.0, -1.0, -1.0, -1.0, -1.0, -1.0, -1.0, -1.0, -1.0, -1.0, -1.0, -1.0, -1.0, -1.0, -1.0, -1.0], [-1.0, -1.0, -1.0, -1.0, -1.0, -1.0, -1.0, -1.0, -1.0, -1.0, -1.0, -1.0, -1.0, -1.0, -1.0, -1.0, -1.0, -1.0, -1.0, -1.0, -1.0, -1.0, -1.0, -1.0, -1.0, -1.0, -1.0], [-1.0, -1.0, -1.0, -1.0, -1.0, -1.0, -1.0, -1.0, -1.0, -1.0, -1.0, -1.0, -1.0, -1.0, -1.0, -1.0, -1.0, -1.0, -1.0, -1.0, -1.0, -1.0, -1.0, -1.0, -1.0, -1.0, -1.0], [-1.0, -1.0, -1.0, -1.0, -1.0, -1.0, -1.0, -1.0, -1.0, -1.0, -1.0, -1.0, -1.0, -1.0, -1.0, -1.0, -1.0, -1.0, -1.0, -1.0, -1.0, -1.0, -1.0, -1.0, -1.0, -1.0, -1.0], [-1.0, -1.0, -1.0, -1.0, -1.0, -1.0, -1.0, -1.0, -1.0, -1.0, -1.0, -1.0, -1.0, -1.0, -1.0, -1.0, -1.0, -1.0, -1.0, -1.0, -1.0, -1.0, -1.0, -1.0, -1.0, -1.0, -1.0], [-1.0, -1.0, -1.0, -1.0, -1.0, -1.0, -1.0, -1.0, -1.0, -1.0, -1.0, -1.0, -1.0, 728.0, -1.0, -1.0, -1.0, -1.0, -1.0, -1.0, -1.0, -1.0, -1.0, -1.0, -1.0, -1.0, -1.0], [-1.0, -1.0, -1.0, -1.0, -1.0, -1.0, -1.0, -1.0, -1.0, -1.0, -1.0, -1.0, -1.0, -1.0, -1.0, -1.0, -1.0, -1.0, -1.0, -1.0, -1.0, -1.0, -1.0, -1.0, -1.0, -1.0, -1.0], [-1.0, -1.0, -1.0, -1.0, -1.0, -1.0, -1.0, -1.0, -1.0, -1.0, -1.0, -1.0, -1.0, -1.0, -1.0, -1.0, -1.0, -1.0, -1.0, -1.0, -1.0, -1.0, -1.0, -1.0, -1.0, -1.0, -1.0], [-1.0, -1.0, -1.0, -1.0, -1.0, -1.0, -1.0, -1.0, -1.0, -1.0, -1.0, -1.0, -1.0, -1.0, -1.0, -1.0, -1.0, -1.0, -1.0, -1.0, -1.0, -1.0, -1.0, -1.0, -1.0, -1.0, -1.0], [-1.0, -1.0, -1.0, -1.0, -1.0, -1.0, -1.0, -1.0, -1.0, -1.0, -1.0, -1.0, -1.0, -1.0, -1.0, -1.0, -1.0, -1.0, -1.0, -1.0, -1.0, -1.0, -1.0, -1.0, -1.0, -1.0, -1.0], [-1.0, -1.0, -1.0, -1.0, -1.0, -1.0, -1.0, -1.0, -1.0, -1.0, -1.0, -1.0, -1.0, -1.0, -1.0, -1.0, -1.0, -1.0, -1.0, -1.0, -1.0, -1.0, -1.0, -1.0, -1.0, -1.0, -1.0], [-1.0, -1.0, -1.0, -1.0, -1.0, -1.0, -1.0, -1.0, -1.0, -1.0, -1.0, -1.0, -1.0, -1.0, -1.0, -1.0, -1.0, -1.0, -1.0, -1.0, -1.0, -1.0, -1.0, -1.0, -1.0, -1.0, -1.0], [-1.0, -1.0, -1.0, -1.0, -1.0, -1.0, -1.0, -1.0, -1.0, -1.0, -1.0, -1.0, -1.0, -1.0, -1.0, -1.0, -1.0, -1.0, -1.0, -1.0, -1.0, -1.0, -1.0, -1.0, -1.0, -1.0, -1.0], [-1.0, -1.0, -1.0, -1.0, -1.0, -1.0, -1.0, -1.0, -1.0, -1.0, -1.0, -1.0, -1.0, -1.0, -1.0, -1.0, -1.0, -1.0, -1.0, -1.0, -1.0, -1.0, -1.0, -1.0, -1.0, -1.0, -1.0], [-1.0, -1.0, -1.0, -1.0, -1.0, -1.0, -1.0, -1.0, -1.0, -1.0, -1.0, -1.0, -1.0, -1.0, -1.0, -1.0, -1.0, -1.0, -1.0, -1.0, -1.0, -1.0, -1.0, -1.0, -1.0, -1.0, -1.0], [-1.0, -1.0, -1.0, -1.0, -1.0, -1.0, -1.0, -1.0, -1.0, -1.0, -1.0, -1.0, -1.0, -1.0, -1.0, -1.0, -1.0, -1.0, -1.0, -1.0, -1.0, -1.0, -1.0, -1.0, -1.0, -1.0, -1.0], [-1.0, -1.0, -1.0, -1.0, -1.0, -1.0, -1.0, -1.0, -1.0, -1.0, -1.0, -1.0, -1.0, -1.0, -1.0, -1.0, -1.0, -1.0, -1.0, -1.0, -1.0, -1.0, -1.0, -1.0, -1.0, -1.0, -1.0], [-1.0, -1.0, -1.0, -1.0, -1.0, -1.0, -1.0, -1.0, -1.0, -1.0, -1.0, -1.0, -1.0, -1.0, -1.0, -1.0, -1.0, -1.0, -1.0, -1.0, -1.0, -1.0, -1.0, -1.0, -1.0, -1.0, -1.0], [-1.0, -1.0, -1.0, -1.0, -1.0, -1.0, -1.0, -1.0, -1.0, -1.0, -1.0, -1.0, -1.0, -1.0, -1.0, -1.0, -1.0, -1.0, -1.0, -1.0, -1.0, -1.0, -1.0, -1.0, -1.0, -1.0, -1.0]], "Divider (kernel sum)"=sgl 10.0 ("Divider"), "error in (no error)"=w255, "Image Src"=w252) -> ("error out"=w265:errorcluster, "Image Dst Out"=w264:T9)  [unwired: 3 in, 3 out]
            n54 = case shown="\"Range 1\", Default" w236 {
              tunnel: ["Range 1 Templates - RIGHT" "Range 0 Templates" "Range 2 Templates" "Range 3 Templates"] -> w295
              tunnel: [w686 w693 w705 w712] -> w293
              tunnel: [sgl 2.0 sgl 0.0 sgl 5.0 sgl 5.0] -> w292
              tunnel: [1 1 3 3] -> w291
              tunnel: [w683 w697 w701 w710] -> w238
              tunnel: "Correlation Score Threhsold" -> [w683 _ w701 w710]
              tunnel: "Correlation Score Threhsold (Range 0)" -> [_ w697 _ _]
              tunnel: [w681 w691 w699 w708] -> w233
              tunnel: [w680 w689 w698 w707] -> w232
              frame "Range 1", Default {
                w687 = TRUE
                w679 = FALSE
                n55 = Unbundle By Name("Range 1 Default\nSetting Values") -> ("Max Scale Diff\nfrom Main"=w681:dbl, "Beacon Cushion (px)"=w680:dbl)
                n56 = Build Array(w679, w679, w679, w687, w687) -> (w686:bool[])
              }
              frame "Range 0" {
                (unwired) TRUE
                w694 = FALSE
                n57 = Unbundle By Name("Range 0 Default\nSetting Values") -> ("Max Scale Diff\nfrom Main"=w691:dbl, "Beacon Cushion (px)"=w689:dbl)
                n58 = Build Array(w694, w694, w694, w694, w694) -> (w693:bool[])
              }
              frame "Range 2" {
                (unwired) FALSE
                w706 = TRUE
                n59 = Unbundle By Name("Range 2 Default\nSetting Values") -> ("Max Scale Diff\nfrom Main"=w699:dbl, "Beacon Cushion (px)"=w698:dbl)
                n60 = Build Array(w706, w706, w706, w706, w706) -> (w705:bool[])
              }
              frame "Range 3" {
                (unwired) FALSE
                w713 = TRUE
                n61 = Unbundle By Name("Range 3 Default\nSetting Values") -> ("Max Scale Diff\nfrom Main"=w708:dbl, "Beacon Cushion (px)"=w707:dbl)
                n62 = Build Array(w713, w713, w713, w713, w713) -> (w712:bool[])
              }
            }
            n63 = Unbundle(w295) -> ("Sub - 2 File Path"=w249:path, "Sub Beacon Template File Path - ARRAY"=w294:path[])
            n64 = call "pattern_match_subvi.vi"("Match Image In"=w264, "Settings"=w248, "Template Image In"=w247, "select (false=mod))"="select (true= use advanced features\nfase= dont use)", "ROI Descriptor"=w250, "error in (no error)"=w265, "Path In"=w249) -> ("Refnum out"=w244:T9, "Number of Matches"=w245:i32, "Matches"=w246:T14[], "error out"=w243:errorcluster)  [unwired: 5 in]
            n65 = Equal?(x=w245, y=1) -> (x = y?=w300:bool)
            n66 = Array To Cluster(array=w246) -> (cluster=w299:T15)
            n67 = Unbundle By Name(w299) -> ("Matches[0].Correlation Score"=w298:sgl)
            "Current Correlation Score" <- w298
            n68 = Greater?(x=w298, y=w238) -> (0:w297:bool)
            n69 = And(x=w300, y=w297) -> (x .and. y?=w296:bool)
            n70 = case shown="True" w296 {
              tunnel: w244 -> [w792 w825]
              tunnel: w292 -> [_ w827]
              tunnel: w293 -> [_ w826]
              tunnel: w243 -> [_ w824]
              tunnel: w248 -> [_ w823]
              tunnel: [w797 w813] -> w226
              tunnel: [w796 w822] -> w227
              tunnel: [w796 w821] -> w228
              tunnel: [w796 w806] -> w229
              tunnel: [w796 w820] -> w345
              tunnel: [w795 w811] -> w340
              tunnel: [w795 w812] -> w339
              tunnel: [w792 w819] -> w309
              tunnel: [w793 w815] -> w235
              tunnel: w299 -> [_ w818]
              tunnel: w294 -> [_ w817]
              tunnel: w236 -> [_ w816]
              tunnel: [w789 w814] -> w234
              tunnel: w233 -> [_ w810]
              tunnel: w232 -> [_ w809]
              frame False {
                w794 = 0.0
                w795 = sgl 0.0 ("Scale")
                # "Don't Move servo"
                n71 = Bundle(w794, w794) -> (w793:cluster{dbl, dbl})  [unwired: 1 in]
                n72 = Bundle(159.0, 119.0) -> (w789:cluster{dbl, dbl})  [unwired: 1 in]
                n73 = Initialize Array(FALSE, 5 ("dimension size")) -> (w797:bool[])
                n74 = Initialize Array(0.0, 5 ("dimension size")) -> (w796:dbl[])
              }
              frame True {
                n75 = Unbundle By Name(w818) -> ("Matches[0].Position"=w815:cluster{"x":sgl, "y":sgl}, "Matches[0].Bounding Box"=w828:cluster{"x":sgl, "y":sgl}[], "Matches[0].Scale"=w811:sgl, "Matches[0].Score"=w812:sgl)
                n76 = case shown="\"Range 1\", Default" w816 {
                  tunnel: w828 -> [w872 _]
                  tunnel: w827 -> [w868 _]
                  tunnel: w826 -> [w856 _]
                  tunnel: w825 -> [w854 w927]
                  tunnel: w824 -> [w853 _]
                  tunnel: w823 -> [w852 _]
                  tunnel: [w850 w936] -> w805
                  tunnel: [w849 w930] -> w822
                  tunnel: [w848 w931] -> w821
                  tunnel: [w847 w932] -> w806
                  tunnel: [w846 w933] -> w820
                  tunnel: w811 -> [w845 _]
                  tunnel: [w844 w927] -> w819
                  tunnel: w817 -> [w843 _]
                  tunnel: w811 -> [_ w928]
                  tunnel: [w842 w924] -> w814
                  tunnel: w815 -> [w842 _]
                  tunnel: w809 -> [w841 _]
                  frame "Range 1", Default {
                    # "Build ROI for Individual Beacons Based on Main Bounding Box"
                    # "Starting X Lower Bound"
                    # "Beacons to Search For"
                    # "Length of\nIndividual Beacon ROI"
                    # "Length of Bounding Box"
                    # "Draw Bounding Box on Display Image"
                    n77 = Array To Cluster(array=w872) -> (cluster=w873:T16)
                    n78 = Unbundle By Name(w873) -> ("Bounding Box[0].x"=w866:sgl, "Bounding Box[0].y"=w863:sgl, "Bounding Box[2].x"=w869:sgl, "Bounding Box[2].y"=w862:sgl)
                    n79 = Bundle("x"=w866, "y"=w863, "x"=w869, "y"=w862) -> (w871:cluster{"x":sgl, "y":sgl, "x":sgl, "y":sgl})  [unwired: 1 in]
                    n80 = call "IMAQ Overlay Rectangle"("Rectangle"=w871, "Image"=w854) -> ("Image Out"=w851:T9)  [unwired: 8 in, 1 out]
                    n81 = Subtract(x=w869, y=w866) -> (x-y=w870:sgl)
                    n82 = Divide(x=w870, y=w868) -> (x/y=w867:sgl)
                    n83 = Multiply(x=w841, y=w845) -> (x*y=w864:dbl)
                    n84 = Divide(x=w864, y=sgl 100.0) -> (x/y=w859:dbl)
                    n85 = Subtract(x=w863, y=w859) -> (x-y=w861:dbl)
                    n86 = Add(x=w862, y=w859) -> (x+y=w860:dbl)
                    n87 = for {
                      N: 5 -> [_]
                      tunnel: w856 -> [w919] mode=indexing
                      shift-right: [w913] -> _
                      shift-left: w866 -> [w918]
                      tunnel: w867 -> [w917]
                      tunnel: w861 -> [w910]
                      tunnel: w860 -> [w909]
                      tunnel: [w916] -> w855 mode=indexing
                      tunnel: w859 -> [w911]
                      # "Divide Bounding Box"
                      # "Upper Bound of Current is\nLower Bound for Next"
                      n88 = case shown="True" w919 {
                        tunnel: w918 -> [w920 w921]
                        tunnel: w917 -> [_ w923]
                        tunnel: [w920 w922] -> w913
                        tunnel: [w920 w921] -> w915
                        frame False {
                          # "Don't Care"
                        }
                        frame True {
                          # "X Lower Bound"
                          n89 = Add(x=w921, y=w923) -> (x+y=w922:sgl)
                        }
                      }
                      n90 = Subtract(x=w915, y=w911) -> (x-y=w914:dbl)
                      n91 = Add(x=w913, y=w911) -> (x+y=w912:dbl)
                      n92 = call "Bound_RO_L_R0.vi"("Bottom Right - Y"=w909, "Right - X"=w912, "Top Left - Y"=w910, "Top  Left - x"=w914) -> ("ROI Descriptor"=w916:T12)  [unwired: 7 in]
                    }
                    n93 = for {
                      N: 5 -> [_]
                      tunnel: w854 -> [w886]
                      tunnel: w853 -> [w885]
                      tunnel: w855 -> [w878] mode=indexing
                      tunnel: w843 -> [w884] mode=indexing
                      tunnel: [w883] -> w849 mode=indexing
                      tunnel: [w882] -> w848 mode=indexing
                      tunnel: [w881] -> w850 mode=indexing
                      tunnel: w856 -> [w880] mode=indexing
                      tunnel: w852 -> [w879]
                      shift-right: [w876] -> w844
                      shift-left: w851 -> [w877]
                      tunnel: [w875] -> w847 mode=indexing
                      tunnel: [w874] -> w846 mode=indexing
                      n94 = case shown="True" w880 {
                        tunnel: w886 -> [_ w901]
                        tunnel: w885 -> [_ w900]
                        tunnel: w878 -> [_ w899]
                        tunnel: w884 -> [_ w898]
                        tunnel: [w887 w894] -> w883
                        tunnel: [w887 w893] -> w882
                        tunnel: [FALSE w892] -> w881
                        tunnel: w879 -> [_ w891]
                        tunnel: [w887 w890] -> w875
                        tunnel: [w887 w889] -> w874
                        frame False {
                          w887 = sgl 0.0 ("x")
                        }
                        frame True {
                          n95 = call "Sub Beacon Pattern Match"("Image In"=w901, "ROI Descriptor (Geometric Matching 1)"=w899, "Settings (Geometric Matching 1)"=w891, "Template File Path (Geometric Matching 1)"=w898, "error in"=w900) -> ("Matches (Geometric Matching 1)"=w895:T14[], "Number of Matches (Geometric Matching 1)"=w896:i32)  [unwired: 19 in, 2 out]
                          n96 = Equal?(x=w896, y=1) -> (x = y?=w892:bool)
                          n97 = case shown="True" w892 {
                            tunnel: w895 -> [_ w907]
                            tunnel: [w902 w906] -> w894
                            tunnel: [w902 w905] -> w893
                            tunnel: [w902 w904] -> w890
                            tunnel: [w902 w903] -> w889
                            frame False {
                              w902 = sgl 0.0 ("x")
                            }
                            frame True {
                              n98 = Array To Cluster(array=w907) -> (cluster=w908:T17)
                              n99 = Unbundle By Name(w908) -> ("Matches (Geometric Matching 1)[0].Position.x"=w906:sgl, "Matches (Geometric Matching 1)[0].Position.y"=w905:sgl, "Matches (Geometric Matching 1)[0].Scale"=w904:sgl, "Matches (Geometric Matching 1)[0].Score"=w903:sgl)
                            }
                          }
                        }
                      }
                      n100 = call "IMAQ Overlay ROI"("ROI Descriptor"=w878, "Image"=w877) -> ("Image Out"=w876:T9)  [unwired: 8 in, 1 out]
                    }
                    "Horiztonall Beacon \nCushion (pixels)" <- w841
                  }
                  frame "Range 0" {
                    w929 = sgl 0.0
                    w935 = FALSE
                    # "Don't Move servo"
                    # "Insert Current Scale into index 0"
                    n101 = Bundle(159.0, 119.0) -> (w924:cluster{dbl, dbl})  [unwired: 1 in]
                    n102 = Build Array(TRUE, w935, w935, w935, w935) -> (w936:bool[])
                    n103 = Build Array(w928, w929, w929, w929, w929) -> (w932:sgl[])
                    n104 = Build Array(w929, w929, w929, w929, w929) -> (w931:sgl[])
                    n105 = Build Array(w929, w929, w929, w929, w929) -> (w933:sgl[])
                    n106 = Build Array(w929, w929, w929, w929, w929) -> (w930:sgl[])
                  }
                }
                n107 = Boolean To (0,1)(Boolean=w805) -> (0, 1=w804:i16[])
                n108 = Add Array Elements(numeric array=w804) -> (sum=w803:i16)
                n109 = Add Array Elements(numeric array=w806) -> (sum=w808:sgl)
                n110 = Divide(x=w808, y=w803) -> (x/y=w807:sgl)
                n111 = for {
                  N: 5 -> [_]
                  tunnel: w807 -> [w833]
                  tunnel: w805 -> [w832] mode=indexing
                  tunnel: [w831] -> w813 mode=indexing
                  tunnel: w806 -> [w830] mode=indexing
                  tunnel: w810 -> [w829]
                  # "Check if Scale is within threshold of main,\ndsicard if not"
                  n112 = case shown="True" w832 {
                    selector: w832 -> [w834 _]
                    tunnel: w830 -> [_ w840]
                    tunnel: w833 -> [_ w839]
                    tunnel: [w834 w836] -> w831
                    tunnel: w829 -> [_ w835]
                    frame False {
                    }
                    frame True {
                      n113 = Subtract(x=w840, y=w839) -> (x-y=w838:sgl)
                      n114 = Absolute Value(x=w838) -> (abs(x)=w837:sgl)
                      n115 = Less?(x=w837, y=w835) -> (x < y?=w836:bool)
                    }
                  }
                }
              }
            }
            "Beacons Found" <- w226
            "X Coordinates" <- w227
            "Y Coordinates" <- w228
            "Beacon - Scales" <- w229
            "beacon - Scores" <- w345
            "Current  Scale" <- w340
            "Current  Score" <- w339
            n116 = shared-variable "RT myRIO Target - Overlord\\Localization_Variables_r0.lvlib\\RIGHT_BEACON_Scales"(w229) -> ()  [unwired: 1 in, 1 out]
            n117 = shared-variable "RT myRIO Target - Overlord\\Localization_Variables_r0.lvlib\\RIGHT_BEACON_X_array"(w227) -> ()  [unwired: 1 in, 1 out]
            n118 = shared-variable "RT myRIO Target - Overlord\\Localization_Variables_r0.lvlib\\RIGHT_BEACON_Y_array"(w228) -> ()  [unwired: 1 in, 1 out]
            n119 = shared-variable "RT myRIO Target - Overlord\\Localization_Variables_r0.lvlib\\RIGHT_BEACON_BOOL_array"(w226) -> ()  [unwired: 1 in, 1 out]
            n120 = Boolean To (0,1)(Boolean=w226) -> (0, 1=w347:i16[])
            n121 = Add Array Elements(numeric array=w347) -> (sum=w346:i16)
            n122 = Greater Or Equal?(x=w346, y=w291) -> (x >= y?=w282:bool)
            "Current Valid?" <- w282
            n123 = local read "History Size"() -> (w331:i32)
            n124 = Decrement(x=w331) -> (x-1=w344:i32)
            n125 = for {
              N: w331 -> [_]
              shift-right: [w767] -> w302
              shift-left: w343 -> [w755]
              tunnel: w344 -> [w763]
              shift-right: [w760] -> w270
              shift-left: w342 -> [w762]
              shift-right: [w759] -> w301
              shift-left: w341 -> [w761]
              tunnel: w340 -> [w758]
              tunnel: w339 -> [w757]
              tunnel: w282 -> [w756]
              i -> [w766]
              # "Reverse Index"
              n126 = Subtract(x=w763, y=w766) -> (x-y=w764:i32)
              n127 = Equal To 0?(x=w764) -> (x = 0?=w765:bool)
              n128 = case shown="True" w765 {
                tunnel: w764 -> [w768 w787]
                tunnel: w755 -> [w778 w780]
                tunnel: [w776 w779] -> w767
                tunnel: w756 -> [_ w788]
                tunnel: w762 -> [w773 w786]
                tunnel: w761 -> [w772 w785]
                tunnel: [w771 w783] -> w760
                tunnel: [w770 w784] -> w759
                tunnel: w758 -> [_ w782]
                tunnel: w757 -> [_ w781]
                frame False {
                  # "Shift Old"
                  n129 = Decrement(x=w768) -> (x-1=w769:i32)
                  n130 = Index Array(array=w778, index=w769) -> (element=w777:bool)
                  n131 = Index Array(array=w773, index=w769) -> (element=w775:dbl)
                  n132 = Index Array(array=w772, index=w769) -> (element=w774:dbl)
                  n133 = Replace Array Subset(array=w778, new element=w777, index=w768) -> (w776:bool[])
                  n134 = Replace Array Subset(array=w773, new element=w775, index=w768) -> (w771:dbl[])
                  n135 = Replace Array Subset(array=w772, new element=w774, index=w768) -> (w770:dbl[])
                }
                frame True {
                  # "Score"
                  # "Scale"
                  # "Valid"
                  # "insert New"
                  n136 = Replace Array Subset(array=w786, new element=w782, index=w787) -> (w783:dbl[])
                  n137 = Replace Array Subset(array=w785, new element=w781, index=w787) -> (w784:dbl[])
                  n138 = Replace Array Subset(array=w780, new element=w788, index=w787) -> (w779:bool[])
                }
              }
            }
            n139 = Boolean To (0,1)(Boolean=w302) -> (0, 1=w337:i16[])
            n140 = Add Array Elements(numeric array=w337) -> (sum=w336:i16)
            n141 = Greater Or Equal?(x=w336, y="Valid Treshold\nfor Lock") -> (x >= y?=w230:bool)
            "Lock Status" <- w230
            n142 = shared-variable "RT myRIO Target - Overlord\\Localization_Variables_r0.lvlib\\Image Lock - R"(w230) -> ()  [unwired: 1 in, 1 out]
            n143 = Initialize Array(u8 0, "Max Window\n for Avg") -> (w334:u8[])
            n144 = while {
              shift-right: [w738] -> w330
              shift-left: w334 -> [w740]
              tunnel: w302 -> [w746] mode=indexing
              shift-right: [w744] -> w327
              shift-left: u8 0 -> [w747]
              tunnel: w331 -> [w745]
              tunnel: "Max Window\n for Avg" -> [w737]
              i -> [w739]
              stop <- w741 stop-if-true
              # "Grab Last 'X' Valid Indexes"
              n145 = case shown="True" w746 {
                tunnel: w747 -> [w749 w751]
                tunnel: [w749 w754] -> w744
                tunnel: w740 -> [w748 w753]
                tunnel: w739 -> [_ w752]
                tunnel: [w748 w750] -> w738
                frame False {
                }
                frame True {
                  # "Update Index\nto use"
                  # "Increment\nValid Count"
                  n146 = Replace Array Subset(array=w753, new element=w752, index=w751) -> (w750:u8[])
                  n147 = Increment(x=w751) -> (x+1=w754:u8)
                }
              }
              n148 = Greater?(x=w739, y=w745) -> (0:w742:bool)
              n149 = Greater Or Equal?(x=w744, y=w737) -> (x >= y?=w743:bool)
              n150 = Or(x=w743, y=w742) -> (x .or. y?=w741:bool)
            }
            n151 = Greater Or Equal?(x=w327, y=u8 2) -> (x >= y?=w328:bool)
            n152 = case shown="True" w328 {
              tunnel: w327 -> [_ w721]
              tunnel: w330 -> [_ w727]
              tunnel: w270 -> [_ w726]
              tunnel: w301 -> [_ w725]
              tunnel: ["Avg Scale - Last" w719] -> w290
              tunnel: ["Avg Score - Last" w718] -> w289
              frame False {
              }
              frame True {
                w724 = 0.0
                n153 = for {
                  N: w721 -> [_]
                  tunnel: w727 -> [w734] mode=indexing
                  tunnel: w726 -> [w736]
                  tunnel: w725 -> [w735]
                  shift-right: [w732] -> w723
                  shift-left: w724 -> [w730]
                  shift-right: [w733] -> w722
                  shift-left: w724 -> [w729]
                  # "Fetch Last Valid Values"
                  n154 = Index Array(array=w736, index=w734) -> (element=w731:dbl)
                  n155 = Index Array(array=w735, index=w734) -> (element=w728:dbl)
                  n156 = Add(x=w731, y=w730) -> (x+y=w732:dbl)
                  n157 = Add(x=w728, y=w729) -> (x+y=w733:dbl)
                }
                n158 = To Double Precision Float(number=w721) -> (double precision float=w720:dbl)
                n159 = Divide(x=w723, y=w720) -> (x/y=w719:dbl)
                n160 = Divide(x=w722, y=w720) -> (x/y=w718:dbl)
                n161 = local write "Avg Scale - Last"(w719) -> ()
                n162 = local write "Avg Score - Last"(w718) -> ()
              }
            }
            "Avg Score" <- w289
            "Avg Scale" <- w290
            n163 = And(x=w230, y=w268) -> (x .and. y?=w269:bool)
            n164 = case shown="False" w269 {
              selector: w269 -> [_ w351]
              tunnel: [w349 w350] -> w267
              tunnel: w268 -> [w349 _]
              frame False {
              }
              frame True {
                # "Pull Down Start Up \nFlag"
                n165 = Not(x=w351) -> (.not. x?=w350:bool)
              }
            }
            n166 = Unbundle By Name(w248) -> ("Minimum Match Score"=w287:sgl, "Range Settings"=w314:T7[], "Curve Parameters"=w284:T6)
            n167 = Index Array(array=w314, index=u32 1) -> (element=w315:T7)
            n168 = Unbundle(w315) -> ("Min"=w286:dbl, "Max"=w285:dbl)  [unwired: 1 out]
            n169 = case shown="False" w267 {
              tunnel: w230 -> [w374 _]
              tunnel: w236 -> [w373 w678]
              tunnel: w290 -> [w372 _]
              tunnel: [w356 w678] -> w272
              tunnel: w290 -> [w371 _]
              tunnel: w289 -> [w370 _]
              tunnel: "Score\nCushion" -> [w369 _]
              tunnel: w287 -> [w368 w675]
              tunnel: w286 -> [w367 w674]
              tunnel: w285 -> [w366 w673]
              tunnel: w235 -> [w365 _]
              tunnel: w250 -> [w364 w677]
              tunnel: w284 -> [w363 _]
              tunnel: w284 -> [w362 w676]
              tunnel: [w361 w675] -> w276
              tunnel: [w360 w674] -> w274
              tunnel: [w359 w673] -> w275
              tunnel: [w358 w677] -> w273
              tunnel: [w357 w676] -> w281
              tunnel: [w355 FALSE] -> w283
              tunnel: w282 -> [w354 _]
              tunnel: w270 -> [w353 w671]
              tunnel: [w352 w671] -> w271
              frame False {
                # "Current Template"
                # "Image Lock?"
                n170 = case shown="False" w374 {
                  tunnel: w373 -> [_ w466]
                  tunnel: [w376 w429] -> w356
                  tunnel: w372 -> [_ w467]
                  tunnel: w371 -> [_ w465]
                  tunnel: w370 -> [_ w463]
                  tunnel: w369 -> [_ w462]
                  tunnel: w368 -> [_ w461]
                  tunnel: w367 -> [_ w460]
                  tunnel: w366 -> [_ w459]
                  tunnel: w365 -> [_ w458]
                  tunnel: w364 -> [_ w457]
                  tunnel: w363 -> [_ w454]
                  tunnel: w362 -> [w381 w439]
                  tunnel: [w380 w434] -> w357
                  tunnel: [w392 w433] -> w358
                  tunnel: [w401 w432] -> w361
                  tunnel: [w400 w431] -> w360
                  tunnel: [w399 w430] -> w359
                  tunnel: [FALSE w428] -> w355
                  tunnel: w354 -> [_ w427]
                  tunnel: w353 -> [w378 w426]
                  tunnel: [w378 w425] -> w352
                  frame False {
                    # "Apply default settings for the selected template"
                    # "Initial ROI Descriptor"
                    # "Check Other Camera?"
                    n171 = shared-variable "RT myRIO Target - Overlord\\Localization_Variables_r0.lvlib\\Image Lock - L"() -> (w375:bool)  [unwired: 1 in, 1 out]
                    n172 = case shown="True" w375 {
                      tunnel: [w407 w424] -> w376
                      frame False {
                        # "No Lock Available, Choose Based off last position"
                        n173 = shared-variable "RT myRIO Target - Overlord\\Localization_Variables_r0.lvlib\\Last Robot Position"() -> (w406:cluster{"X":sgl, "Y":sgl})  [unwired: 1 in, 1 out]
                        n174 = Unbundle By Name(w406) -> ("X"=w408:sgl)
                        n175 = Less?(x=w408, y=sgl 3.0) -> (x < y?=w409:bool)
                        n176 = case shown="False" w409 {
                          tunnel: [w412 T4."Range 0" ("Current Template")] -> w407
                          tunnel: w408 -> [w411 _]
                          frame False {
                            n177 = Less?(x=w411, y=sgl 5.0) -> (x < y?=w413:bool)
                            n178 = case shown="True" w413 {
                              tunnel: [w416 T4."Range 1" ("Current Template")] -> w412
                              tunnel: w411 -> [w418 _]
                              frame False {
                                n179 = Less?(x=w418, y=sgl 10.0) -> (x < y?=w415:bool)
                                n180 = case shown="False" w415 {
                                tunnel: [T4."Range 3" ("Current Template") T4."Range 2" ("Current Template")] -> w416
                                frame False {
                                }
                                frame True {
                                }
                                }
                              }
                              frame True {
                              }
                            }
                          }
                          frame True {
                          }
                        }
                      }
                      frame True {
                        # "If other Camera is Locked, Use its template and apply default settings for that template"
                        n181 = shared-variable "RT myRIO Target - Overlord\\Localization_Variables_r0.lvlib\\Info - Left"() -> (w423:T5)  [unwired: 1 in, 1 out]
                        n182 = Unbundle By Name(w423) -> ("Current Template"=w424:T4)
                      }
                    }
                    n183 = case shown="\"Range 2\"" w376 {
                      tunnel: [w402 w403 w404 w405] -> w377
                      frame "Range 1", Default {
                        n184 = local read "Range 1 Default\nSetting Values"() -> (w402:T1)
                      }
                      frame "Range 2" {
                        n185 = local read "Range 2 Default\nSetting Values"() -> (w403:T1)
                      }
                      frame "Range 3" {
                        n186 = local read "Range 3 Default\nSetting Values"() -> (w404:T1)
                      }
                      frame "Range 0" {
                        n187 = local read "Range 0 Default\nSetting Values"() -> (w405:T1)
                      }
                    }
                    n188 = Unbundle By Name(w377) -> ("Min Score"=w401:dbl, "Min Scale"=w400:dbl, "Max Scale"=w399:dbl, "Curve Parameters"=w382:T18)
                    n189 = Bundle(0, 0, 640, 480, 0) -> (w398:cluster{i32, i32, i32, i32, i32})  [unwired: 1 in]
                    n190 = call "IMAQ Convert Rectangle to ROI"("Rectangle"=w398) -> ("ROI Descriptor"=w392:T12)  [unwired: 8 in, 1 out]
                    n191 = Unbundle By Name(w382) -> ("Min Length"=w386:i32, "Row Search Step"=w387:i32, "Col Search Step"=w388:i32)
                    n192 = Unbundle(w381) -> ("Extraction Mode"=w383:u32, "Edge Threshold"=w384:i32, "Edge Filter Size"=w385:u32, "Max Endpoint Gap"=w389:i32, "Closed"=w390:bool, "Subpixel"=w391:bool)  [unwired: 3 out]
                    n193 = Bundle("Extraction Mode"=w383, "Edge Threshold"=w384, "Edge Filter Size"=w385, "Min Length"=w386, "Row Search Step"=w387, "Col Search Step"=w388, "Max Endpoint Gap"=w389, "Closed"=w390, "Subpixel"=w391) -> (w380:T19)  [unwired: 1 in]
                  }
                  frame True {
                    # "Update Search Settings"
                    # "Next State"
                    # "Changing Templates?"
                    # "Update Template"
                    n194 = case shown="\"Range 1\", Default" w466 {
                      selector: w466 -> [w603 w634 w652 w667]
                      tunnel: w467 -> [w604 w636 w653 w668]
                      tunnel: [w605 w635 w651 w666] -> w429
                      tunnel: [w619 w625 w645 w660] -> w464
                      tunnel: [w618 w624 w644 w659] -> w456
                      tunnel: [w617 w623 w643 w658] -> w455
                      tunnel: [w616 w626 w649 w664] -> w450
                      tunnel: [w615 w628 w646 w661] -> w442
                      tunnel: [w614 w629 w647 w662] -> w441
                      tunnel: [w613 w632 w648 w663] -> w440
                      frame "Range 1", Default {
                        # "Next Template"
                        # "Next Template"
                        n195 = local read "Range 1 Default\nSetting Values"() -> (w620:T1)
                        n196 = Unbundle By Name(w620) -> ("Lower Transition Scale"=w601:sgl, "Upper Transition Scale"=w602:sgl, "ROI Vertical"=w617:dbl, "ROI Horizontal"=w618:dbl, "Scale Cushion"=w619:dbl, "Curve Parameters"=w616:T18, "Min Score"=w615:dbl, "Min Scale"=w614:dbl, "Max Scale"=w613:dbl)
                        n197 = Less?(x=w604, y=w601) -> (x < y?=w612:bool)
                        n198 = Not(x=w612) -> (.not. x?=w611:bool)
                        n199 = Select(t=w603, s=w611, f=T4."Range 2" ("Initial Template 2")) -> (s? t:f=w608:T4)
                        n200 = Greater?(x=w604, y=w602) -> (0:w610:bool)
                        n201 = Not(x=w610) -> (.not. x?=w609:bool)
                        n202 = Select(t=w608, s=w609, f=T4."Range 0" ("Initial Template 2")) -> (s? t:f=w605:T4)
                      }
                      frame "Range 2" {
                        # "Next Template"
                        # "Next Template"
                        n203 = local read "Range 2 Default\nSetting Values"() -> (w633:T1)
                        n204 = Unbundle By Name(w633) -> ("Lower Transition Scale"=w631:sgl, "Upper Transition Scale"=w630:sgl, "ROI Vertical"=w623:dbl, "ROI Horizontal"=w624:dbl, "Scale Cushion"=w625:dbl, "Curve Parameters"=w626:T18, "Min Score"=w628:dbl, "Min Scale"=w629:dbl, "Max Scale"=w632:dbl)
                        n205 = Less?(x=w636, y=w631) -> (x < y?=w640:bool)
                        n206 = Not(x=w640) -> (.not. x?=w639:bool)
                        n207 = Select(t=w634, s=w639, f=T4."Range 3" ("Initial Template 2")) -> (s? t:f=w627:T4)
                        n208 = Greater?(x=w636, y=w630) -> (0:w638:bool)
                        n209 = Not(x=w638) -> (.not. x?=w637:bool)
                        n210 = Select(t=w627, s=w637, f=T4."Range 1" ("Initial Template 2")) -> (s? t:f=w635:T4)
                      }
                      frame "Range 3" {
                        # "Next Template"
                        n211 = local read "Range 3 Default\nSetting Values"() -> (w650:T1)
                        n212 = Unbundle By Name(w650) -> ("Upper Transition Scale"=w642:sgl, "ROI Vertical"=w643:dbl, "ROI Horizontal"=w644:dbl, "Scale Cushion"=w645:dbl, "Curve Parameters"=w649:T18, "Min Score"=w646:dbl, "Min Scale"=w647:dbl, "Max Scale"=w648:dbl)  [unwired: 1 out]
                        n213 = Greater?(x=w653, y=w642) -> (0:w655:bool)
                        n214 = Not(x=w655) -> (.not. x?=w654:bool)
                        n215 = Select(t=w652, s=w654, f=T4."Range 2" ("Initial Template 2")) -> (s? t:f=w651:T4)
                      }
                      frame "Range 0" {
                        # "Next Template"
                        n216 = local read "Range 0 Default\nSetting Values"() -> (w665:T1)
                        n217 = Unbundle By Name(w665) -> ("Lower Transition Scale"=w656:sgl, "ROI Vertical"=w658:dbl, "ROI Horizontal"=w659:dbl, "Scale Cushion"=w660:dbl, "Curve Parameters"=w664:T18, "Min Score"=w661:dbl, "Min Scale"=w662:dbl, "Max Scale"=w663:dbl)  [unwired: 1 out]
                        n218 = Less?(x=w668, y=w656) -> (x < y?=w670:bool)
                        n219 = Not(x=w670) -> (.not. x?=w669:bool)
                        n220 = Select(t=w667, s=w669, f=T4."Range 1" ("Initial Template 2")) -> (s? t:f=w666:T4)
                      }
                    }
                    n221 = Unbundle By Name(w450) -> ("Min Length"=w449:i32, "Row Search Step"=w448:i32, "Col Search Step"=w447:i32)
                    n222 = Unbundle(w454) -> ("Extraction Mode"=w453:u32, "Edge Threshold"=w452:i32, "Edge Filter Size"=w451:u32, "Max Endpoint Gap"=w446:i32, "Closed"=w445:bool, "Subpixel"=w444:bool)  [unwired: 3 out]
                    n223 = Bundle("Extraction Mode"=w453, "Edge Threshold"=w452, "Edge Filter Size"=w451, "Min Length"=w449, "Row Search Step"=w448, "Col Search Step"=w447, "Max Endpoint Gap"=w446, "Closed"=w445, "Subpixel"=w444) -> (w443:T19)  [unwired: 1 in]
                    n224 = Not Equal?(x=w429, y=w466) -> (x != y?=w428:bool)
                    n225 = case shown="True" w428 {
                      tunnel: w427 -> [w490 _]
                      tunnel: w465 -> [w489 _]
                      tunnel: w464 -> [w488 _]
                      tunnel: w463 -> [w487 _]
                      tunnel: w462 -> [w486 _]
                      tunnel: w461 -> [w485 _]
                      tunnel: w460 -> [w484 _]
                      tunnel: w459 -> [w483 _]
                      tunnel: w458 -> [w482 _]
                      tunnel: w457 -> [w481 _]
                      tunnel: w456 -> [w480 _]
                      tunnel: w455 -> [w479 _]
                      tunnel: [w477 w564] -> w432
                      tunnel: w443 -> [w468 _]
                      tunnel: [w476 w563] -> w431
                      tunnel: [w475 w562] -> w430
                      tunnel: w442 -> [_ _]
                      tunnel: w441 -> [_ _]
                      tunnel: w440 -> [_ _]
                      tunnel: w429 -> [_ w566]
                      tunnel: w439 -> [_ w579]
                      tunnel: [w469 w578] -> w434
                      tunnel: [w474 w573] -> w438
                      tunnel: [w473 w572] -> w437
                      tunnel: [w472 w556] -> w436
                      tunnel: [w471 w557] -> w435
                      tunnel: w426 -> [w470 w559]
                      tunnel: [w470 w558] -> w425
                      frame False {
                        w478 = 500.0 ("y")
                        # "Current Valid?"
                        # "********"
                        # "Apply Limit to Score"
                        # "Score out"
                        # "Apply Limits to ROI"
                        n226 = case shown="False" w490 {
                          tunnel: w487 -> [_ w539]
                          tunnel: w486 -> [_ w538]
                          tunnel: w489 -> [_ w529]
                          tunnel: w488 -> [w518 w537]
                          tunnel: [w501 w532] -> w474
                          tunnel: [w500 w528] -> w473
                          tunnel: [w499 w531] -> w472
                          tunnel: [w498 w530] -> w471
                          tunnel: [w514 w527] -> w491
                          tunnel: [w513 w526] -> w476
                          tunnel: [w512 w525] -> w475
                          tunnel: w481 -> [w510 _]
                          tunnel: w485 -> [w497 _]
                          tunnel: w484 -> [w496 _]
                          tunnel: w483 -> [w495 _]
                          tunnel: w482 -> [_ w524]
                          tunnel: w480 -> [_ w520]
                          tunnel: w479 -> [_ w521]
                          tunnel: [w493 w519] -> w469
                          tunnel: w468 -> [w493 w519]
                          frame False {
                            # "Current Match was Invalid"
                            n227 = Divide(x=w518, y=sgl 3.0) -> (x/y=w516:dbl)
                            n228 = Subtract(x=w496, y=w516) -> (x-y=w513:dbl)
                            n229 = Add(x=w495, y=w516) -> (x+y=w512:dbl)
                            n230 = Subtract(x=w497, y="Score Decay \nFactor 2") -> (x-y=w514:dbl)
                            n231 = call "IMAQ Convert ROI to Rectangle"("ROI Descriptor"=w510) -> ("Rectangle"=w511:T20)  [unwired: 8 in, 1 out]
                            n232 = Unbundle By Name(w511) -> ("Left"=w505:i32, "Top"=w504:i32, "Right"=w503:i32, "Bottom"=w502:i32)
                            n233 = To Long Integer(number="ROI Decay Factor (px)") -> (32bit integer=w507:i32)
                            n234 = Divide(x="ROI Decay Factor (px)", y=sgl 10.0) -> (x/y=w509:dbl)
                            n235 = Subtract(x=w505, y=w507) -> (x-y=w501:i32)
                            n236 = Add(x=w503, y=w507) -> (x+y=w499:i32)
                            n237 = To Long Integer(number=w509) -> (32bit integer=w506:i32)
                            n238 = Subtract(x=w504, y=w506) -> (x-y=w500:i32)
                            n239 = Add(x=w502, y=w506) -> (x+y=w498:i32)
                          }
                          frame True {
                            (unwired) sgl 109.0 ("x")
                            (unwired) sgl 159.0 ("x")
                            # "Current Match was Valid"
                            # "Center of Image"
                            # "Main ROI"
                            # "Horizontal Scale \n(smaller number = smaller ROI)"
                            n240 = Subtract(x=w539, y=w538) -> (x-y=w527:dbl)
                            n241 = case shown="0, Default" "ROBOT STATE\n(fwd, bwd, neither) 2" {
                              tunnel: w529 -> [w544 w549 w554]
                              tunnel: [w543 w545 w550] -> w525
                              tunnel: w537 -> [w541 w548 w553]
                              tunnel: [w542 w546 w551] -> w526
                              frame 0, Default {
                                n242 = Subtract(x=w544, y=w541) -> (x-y=w542:dbl)
                                n243 = Add(x=w541, y=w544) -> (x+y=w543:dbl)
                              }
                              frame 1 {
                                n244 = Subtract(x=w549, y=5.0) -> (x-y=w546:dbl)
                                n245 = Add(x=w548, y=w549) -> (x+y=w545:dbl)
                              }
                              frame -1 {
                                n246 = Subtract(x=w554, y=w553) -> (x-y=w551:dbl)
                                n247 = Add(x=5.0 ("y"), y=w554) -> (x+y=w550:dbl)
                              }
                            }
                            n248 = Unbundle(w524) -> ("x"=w523:dbl, "y"=w522:dbl)
                            n249 = Divide(x=w529, y=w521) -> (x/y=w535:dbl)
                            n250 = Multiply(x=w529, y=w520) -> (x*y=w533:dbl)
                            n251 = Divide(x=w533, y=sgl 2.0) -> (x/y=w536:dbl)
                            n252 = Add(x=w522, y=w535) -> (x+y=w530:dbl)
                            n253 = Subtract(x=w522, y=w535) -> (x-y=w528:dbl)
                            n254 = Subtract(x=w523, y=w536) -> (x-y=w532:dbl)
                            n255 = Add(x=w536, y=w523) -> (x+y=w531:dbl)
                          }
                        }
                        n256 = Greater?(x=w491, y=w478) -> (0:w492:bool)
                        n257 = Select(t=w491, s=w492, f=w478) -> (s? t:f=w477:dbl)
                      }
                      frame True {
                        w569 = sgl 125.0 ("x")
                        w570 = sgl 109.0 ("x")
                        w571 = sgl 159.0 ("x")
                        # "Reset Scale to 100"
                        # "\"Start Scale\""
                        # "Center of Image"
                        # "Main ROI"
                        # "Horizontal Scale \n(smaller number = smaller ROI)"
                        # "Apply New Curve Parameters"
                        # "Next State"
                        # "Changing States - Apply Initial Settings for that State"
                        n258 = local read "History Size"() -> (w560:i32)
                        n259 = case shown="\"Range 3\"" w566 {
                          tunnel: [w594 w596 w598 w600] -> w565
                          tunnel: [50.0 ("Avg Scale - Last") 90.0 ("Avg Scale - Last") 90.0 ("Avg Scale - Last") 90.0 ("Avg Scale - Last")] -> w555
                          frame "Range 1", Default {
                            n260 = local read "Range 1 Default\nSetting Values"() -> (w594:T1)
                          }
                          frame "Range 2" {
                            n261 = local read "Range 2 Default\nSetting Values"() -> (w596:T1)
                          }
                          frame "Range 3" {
                            n262 = local read "Range 3 Default\nSetting Values"() -> (w598:T1)
                          }
                          frame "Range 0" {
                            n263 = local read "Range 0 Default\nSetting Values"() -> (w600:T1)
                          }
                        }
                        n264 = local write "Avg Scale - Last"(w555) -> ()
                        n265 = for {
                          N: w560 -> [_]
                          tunnel: w555 -> [w590]
                          shift-right: [w589] -> w558
                          shift-left: w559 -> [w592]
                          i -> [w591]
                          n266 = Replace Array Subset(array=w592, new element=w590, index=w591) -> (w589:dbl[])
                        }
                        n267 = Unbundle By Name(w565) -> ("Min Score"=w564:dbl, "Min Scale"=w563:dbl, "Max Scale"=w562:dbl, "Curve Parameters"=w561:T18, "ROI Vertical"=w568:dbl, "ROI Horizontal"=w567:dbl)
                        n268 = Unbundle By Name(w561) -> ("Min Length"=w583:i32, "Row Search Step"=w584:i32, "Col Search Step"=w585:i32)
                        n269 = Unbundle(w579) -> ("Extraction Mode"=w580:u32, "Edge Threshold"=w581:i32, "Edge Filter Size"=w582:u32, "Max Endpoint Gap"=w586:i32, "Closed"=w587:bool, "Subpixel"=w588:bool)  [unwired: 3 out]
                        n270 = Bundle("Extraction Mode"=w580, "Edge Threshold"=w581, "Edge Filter Size"=w582, "Min Length"=w583, "Row Search Step"=w584, "Col Search Step"=w585, "Max Endpoint Gap"=w586, "Closed"=w587, "Subpixel"=w588) -> (w578:T19)  [unwired: 1 in]
                        n271 = Divide(x=w569, y=w568) -> (x/y=w576:dbl)
                        n272 = Multiply(x=w569, y=w567) -> (x*y=w574:dbl)
                        n273 = Divide(x=w574, y=sgl 2.0) -> (x/y=w577:dbl)
                        n274 = Add(x=w570, y=w576) -> (x+y=w557:dbl)
                        n275 = Subtract(x=w570, y=w576) -> (x-y=w572:dbl)
                        n276 = Subtract(x=w571, y=w577) -> (x-y=w573:dbl)
                        n277 = Add(x=w577, y=w571) -> (x+y=w556:dbl)
                      }
                    }
                    n278 = call "Bound_RO_R_R0I.vi"("Bottom Right - Y"=w435, "Right - X"=w436, "Top Left - Y"=w437, "Top  Left - x"=w438) -> ("ROI Descriptor"=w433:T12)  [unwired: 7 in]
                  }
                }
              }
              frame True {
              }
            }
            "Next Template" <- w272
            n279 = Less?(x=w276, y="Absolute\nMinimum Score") -> (x < y?=w320:bool)
            n280 = Less?(x=w274, y="Absolute\nMinimum Scale") -> (x < y?=w323:bool)
            n281 = Greater?(x=w275, y="Absolute\nMaximum Scale") -> (0:w326:bool)
            n282 = Greater?(x=w274, y=w275) -> (0:w322:bool)
            n283 = Less?(x=w275, y=w274) -> (x < y?=w325:bool)
            n284 = Select(t="Absolute\nMinimum Score", s=w320, f=w276) -> (s? t:f=w308:dbl)
            "New Min Score" <- w308
            n285 = Or(x=w323, y=w322) -> (x .or. y?=w321:bool)
            n286 = Or(x=w326, y=w325) -> (x .or. y?=w324:bool)
            n287 = Select(t="Absolute\nMinimum Scale", s=w321, f=w274) -> (s? t:f=w307:dbl)
            "New Low Scale" <- w307
            n288 = Select(t="Absolute\nMaximum Scale", s=w324, f=w275) -> (s? t:f=w306:dbl)
            "New high Scale" <- w306
            n289 = Bundle("index"=w313, "Min"=w307, "Max"=w306) -> (w312:cluster{"index":u32, "Min":dbl, "Max":dbl})  [unwired: 1 in]
            n290 = Replace Array Subset(array=w314, new element=w312, index=w313) -> (w311:T7[])
            n291 = Bundle By Name(cluster=w248, "Minimum Match Score"=w308, "Range Settings"=w311, "Curve Parameters"=w281) -> (w310:T8)
            n292 = call "IMAQ Overlay ROI"("ROI Descriptor"=w273, "Image"=w309) -> ("Image Out"=→"Right Image out":T9)  [unwired: 8 in, 1 out]
            n293 = Unbundle By Name(w281) -> ("Min Length"=w280:i32, "Row Search Step Size"=w279:i32, "Col Search Step Size"=w278:i32)
            n294 = Bundle("Min Length"=w280, "Row Search Step Size"=w279, "Col Search Step Size"=w278) -> (w277:T21)  [unwired: 1 in]
            n295 = Bundle("Min Score"=w308, "Min"=w307, "Max"=w306, w277) -> (w305:T22)  [unwired: 1 in]
            n296 = case shown="True" w283 {
              tunnel: w234 -> [w939 w945]
              tunnel: w282 -> [w940 w951]
              tunnel: w226 -> [_ _]
              tunnel: w305 -> [w942 w949]
              tunnel: w230 -> [w941 w952]
              tunnel: w272 -> [w938 w950]
              tunnel: [w937 w948] -> w231
              frame False {
                n297 = Bundle(w941, w940, "Initial Template"=w938, "Position"=w939, w942) -> (w937:T23)  [unwired: 1 in]
              }
              frame True {
                # "Check if Tracking is Available for the Next Template State"
                n298 = local read "Current Template"() -> (w943:T4)
                n299 = Unbundle(w945) -> ("x"=w947:dbl, "y"=w946:dbl)
                n300 = case shown="\"Range 2\"" w950 {
                  tunnel: w947 -> [w957 w966 _ _]
                  tunnel: w946 -> [w953 w965 _ _]
                  tunnel: w945 -> [_ w963 w974 _]
                  tunnel: [w956 w964 w974 w977] -> w944
                  tunnel: w943 -> [w954 w962 _ _]
                  frame "Range 1" {
                    n301 = case shown="\"Range 2\"" w954 {
                      tunnel: w957 -> [w958 w961]
                      tunnel: [w958 w959] -> w955
                      frame "Range 0", Default {
                      }
                      frame "Range 2" {
                        n302 = Add(x=w961, y=-70.0) -> (x+y=w959:dbl)
                      }
                    }
                    n303 = Bundle("x"=w955, "y"=w953) -> (w956:cluster{"x":dbl, "y":dbl})  [unwired: 1 in]
                  }
                  frame "Range 2" {
                    # "Depends on Current State"
                    n304 = case shown="\"Range 3\"" w962 {
                      tunnel: w966 -> [w971 _ _]
                      tunnel: w965 -> [w968 _ _]
                      tunnel: [w967 w972 w973] -> w964
                      tunnel: w963 -> [_ w972 w973]
                      frame "Range 1" {
                        n305 = Add(x=w971, y=70.0) -> (x+y=w969:dbl)
                        n306 = Bundle(w969, "y"=w968) -> (w967:cluster{dbl, "y":dbl})  [unwired: 1 in]
                      }
                      frame "Range 2", Default {
                      }
                      frame "Range 3" {
                      }
                    }
                  }
                  frame "Range 3", Default {
                  }
                  frame "Range 0" {
                    # "Don't Move servo"
                    n307 = Bundle(159.0, 119.0) -> (w977:cluster{dbl, dbl})  [unwired: 1 in]
                  }
                }
                n308 = Bundle(w952, w951, "Initial Template"=w950, "Position"=w944, w949) -> (w948:T23)  [unwired: 1 in]
              }
            }
            "Tracking Info" <- w231
            n309 = shared-variable "RT myRIO Target - Overlord\\Localization_Variables_r0.lvlib\\Info - Right"(w231) -> ()  [unwired: 1 in, 1 out]
          }
          frame #2 {
            n310 = shared-variable "RT myRIO Target - Overlord\\Localization_Variables_r0.lvlib\\Right Servo Angle_Image"(w979) -> ()  [unwired: 1 in, 1 out]
            n311 = shared-variable "RT myRIO Target - Overlord\\Localization_Variables_r0.lvlib\\RIGHT_FLAG"(TRUE ("RIGHT_FLAG")) -> ()  [unwired: 1 in, 1 out]
          }
        }
        "Startup Flag" <- w194
        "Valid Scale History" <- w201
        "Valid Beacon History - in" <- w203
        "Valid Score History" <- w200
        "Current Search Settings" <- w211
        "Current Template" <- w198
      }
    }
    frame #3 {
      n312 = call <vilib>:"IMAQdx Close Camera.vi"("Session In"=w982) -> ()  [unwired: 10 in, 1 out]
    }
  }
